vi "MC_7_13b_JW.vi"() -> ()   [LabVIEW 2011]
uses:
  <vilib>/Utility/file.llb/Read From Spreadsheet File (string).vi
  <vilib>/Utility/inputDevices.llb/keyboardAcquire.vi
  <vilib>/Utility/file.llb/Write To Spreadsheet File (DBL).vi
  <vilib>/Utility/file.llb/Write To Spreadsheet File (string).vi
  <vilib>/regexp/Match Regular Expression.xnode
panel:
  out "New: Temp":dbl
  out "XY Graph-Lin":cluster{dbl[], dbl[]}[](graph)
  out "Lin Vd":dbl
  out "Lin-Vg Array-Used":dbl[](array[numeric])
  out "Lin Id-Used":dbl[](array[numeric])
  out "Rec: Temp":dbl
  out "Comments":string
  out "Folder Index":dbl caption="Length"
  out "Current \nRecord":string[](array[string])
  out "Transformer \nHeaders":string[](array[string])
  out "Current Device ID":string
  out "Column":string
  out "Row":string
  out "Rec: Concentration":dbl
  out "Rec: Solvent":string
  out "Rec: Method":string
  in  "?":T1(tab)
  out "Rec: Material":string
  in  "Treatment Concentration (mM):":dbl=30.0
  in  "Surface Treatment:":string
  in  "# Drops*:":dbl=inf
  in  "Solution Temp (C):":dbl=55.0
  in  "Relative Humidity (%):":dbl=nan
  in  "Room Temp (F):":dbl=nan
  in  "Time (s):":dbl=80.0
  out "Accel (RPM/s):":dbl
  in  "RPM:":dbl=1000.0
  in  "Wait Time (s):":dbl=10.0
  in  "Sample #:":dbl=1.0
  in  "Fabricator:":string="Jeremy"
  in  "Data File":path
  out "Data Folder":path
  in  "Image Folder":path
  out "Image File":path=path "D:/UserData/Desktop/Jeremy/WFU/Research/Programs/VI mods/Image Not Found.png"
  in  "Ramp (s):":dbl=3.0
  in  "Manuel-Dielectric":bool
  in  "Manuel-Length":bool
  out "Calc: VT-Lin":dbl
  out "New: VT-Lin":dbl
  out "Rec: VT-Lin":dbl caption="VT-Lin" format="%#_3g"
  out "Calc: Trap Density-STS":dbl format="%#_4e"
  out "New: Trap Density-STS":dbl format="%#_4e"
  out "Rec: Trap Density-STS":dbl caption="N-Sat (STS)" format="%#_3e"
  out "Calc: Trap Density-VT":dbl format="%#_4e"
  out "New: Trap Density-VT":dbl format="%#_4e"
  out "Rec: Trap Density-VT":dbl caption="N-Sat (VT)" format="%#_3e"
  out "Calc: Mobility-Lin":dbl format="%#_4e"
  out "New: Mobility-Lin":dbl format="%#_4e"
  out "Rec: Mobility-Lin":dbl caption="Mobility-Lin" format="%#_3e"
  out "Calc: Mobility-Sat":dbl format="%#_4e"
  out "Rec: Length":dbl caption="Length" format="%#_3g"
  out "Rec: Width":dbl caption="Width" format="%#_4g"
  out "Rec: Dielectric (d)":dbl caption="Dielectric (d)" format="%#_3g"
  out "XY Graph":cluster{dbl[], dbl[]}[](graph)
  in  "NumPts":dbl=5.0
  in  "Cancel Button":bool
  in  "Next Button":bool
  in  "Previous Button":bool
  in  "Up Button":bool
  in  "Down Button":bool
  out "Data Name:":string
  in  "Save Changes?":bool
  in  "New: Dielectric":dbl
  in  "New: Length":dbl
  in  "New: Width":dbl
  out "New: Mobility-Sat":dbl format="%#_4e"
  in  "Slide":dbl(slide) step=1.0 scale=-14.3..88.0 scale format="%#_1p"
  in  "Blank Button":bool
  in  "Zoom":i16(slide)=-3 scale=-5.0..5.0
  out "Image Out 2":T2(plugin-control)
  out "Image Out":T2(plugin-control)
  in  "Magnification":u16(ring) items=["5x", "10x", "20x", "50x", "80x"]
  out "Total Width":dbl
  out "Distances":dbl[](array[numeric])
  in  "Undo Button":bool
  in  "Remove Button":bool
  out "Rec: Mobility-Sat":dbl caption="Mobility-Sat" format="%#_3e"
  out "Index":string
  out "Image Name":string
  in  "Export":bool
  out "Calc: VT-Sat":dbl
  out "New: VT-Sat":dbl
  in  "Manual-Width":bool caption="Manual"
  out "XY Graph 2":cluster{dbl[], dbl[]}[](graph)
  in  "Next Button 2":bool
  in  "Previous Button 2":bool
  in  "Slide 2":dbl(slide) step=1.0 scale=-1.0..82.0 scale format="%#_1p"
  out "Calc: STS":dbl
  out "New: STS":dbl
  in  "NumPts 2":dbl=5.0 caption="NumPts"
  out "Rec: VT-Sat":dbl caption="VT-Sat" format="%#_3g"
  out "Rec: STS":dbl caption="STS-Sat" format="%#_3g"
  out "Rec: On/Off":dbl caption="On/Off-Sat" format="%#_3e"
  in  "Save Changes? 2":bool
  in  "Save Changes? 3":bool
  out "Date Recorded":string="Date Recorded" caption="Recorded"
  out "Date Created":string caption="Fabricated"
  out "String":string
  in  "No Image":path=path "D:/UserData/Desktop/Jeremy/WFU/Research/Programs/VI mods/Image Not Found.png"
  in  "Project":path=path "D:/UserData/Desktop/Jeremy/WFU/Research/Programs/Mega Awesome/DeviceData.opj"
  out "Index 2":dbl
  out "Sat Id-Log-Used":dbl[](array[numeric])
  out "Vg Array-Log-Used":dbl[](array[numeric])
  out "ROI Descriptor out":T3 {"Contours"."Type" items=["No Selection", "Point", "Line", "Rectangle", "Oval", "Polygon", "Freehand Region", "Annulus", "Unused2", "Unused3", "Broken Line", "Freehand Line", "Rotated Rectangle"]}
  out "ROI Descriptor":T3 {"Contours"."Type" items=["No Selection", "Point", "Line", "Rectangle", "Oval", "Polygon", "Freehand Region", "Annulus", "Unused2", "Unused3", "Broken Line", "Freehand Line", "Rotated Rectangle"]}
  out "Numeric 3":dbl
  out "Array 6":dbl[][](array[numeric])
  out "Cluster":T4
  out "Array 5":dbl[](array[numeric])
  out "Array 4":dbl[](array[numeric])
  out "Array 3":dbl[](array[numeric])
  out "Numeric 2":dbl
  out "Numeric":dbl
  out "Sat Id-Used":dbl[](array[numeric])
  out "Sat Vg Array-Used":dbl[](array[numeric])
  out "MobVi Index":dbl
  in  "Row Start":dbl=20.0
  # "Data Locations"
  # "Data Location"
  # "Image Location"
  # "Sample Properties"
  # "*     Inf = Full coverage\n   NaN = Unknown or Not Applicable"
  # "Recorded"
  # "Calculated"
  # "Re-Calculated"
  # "Manual"
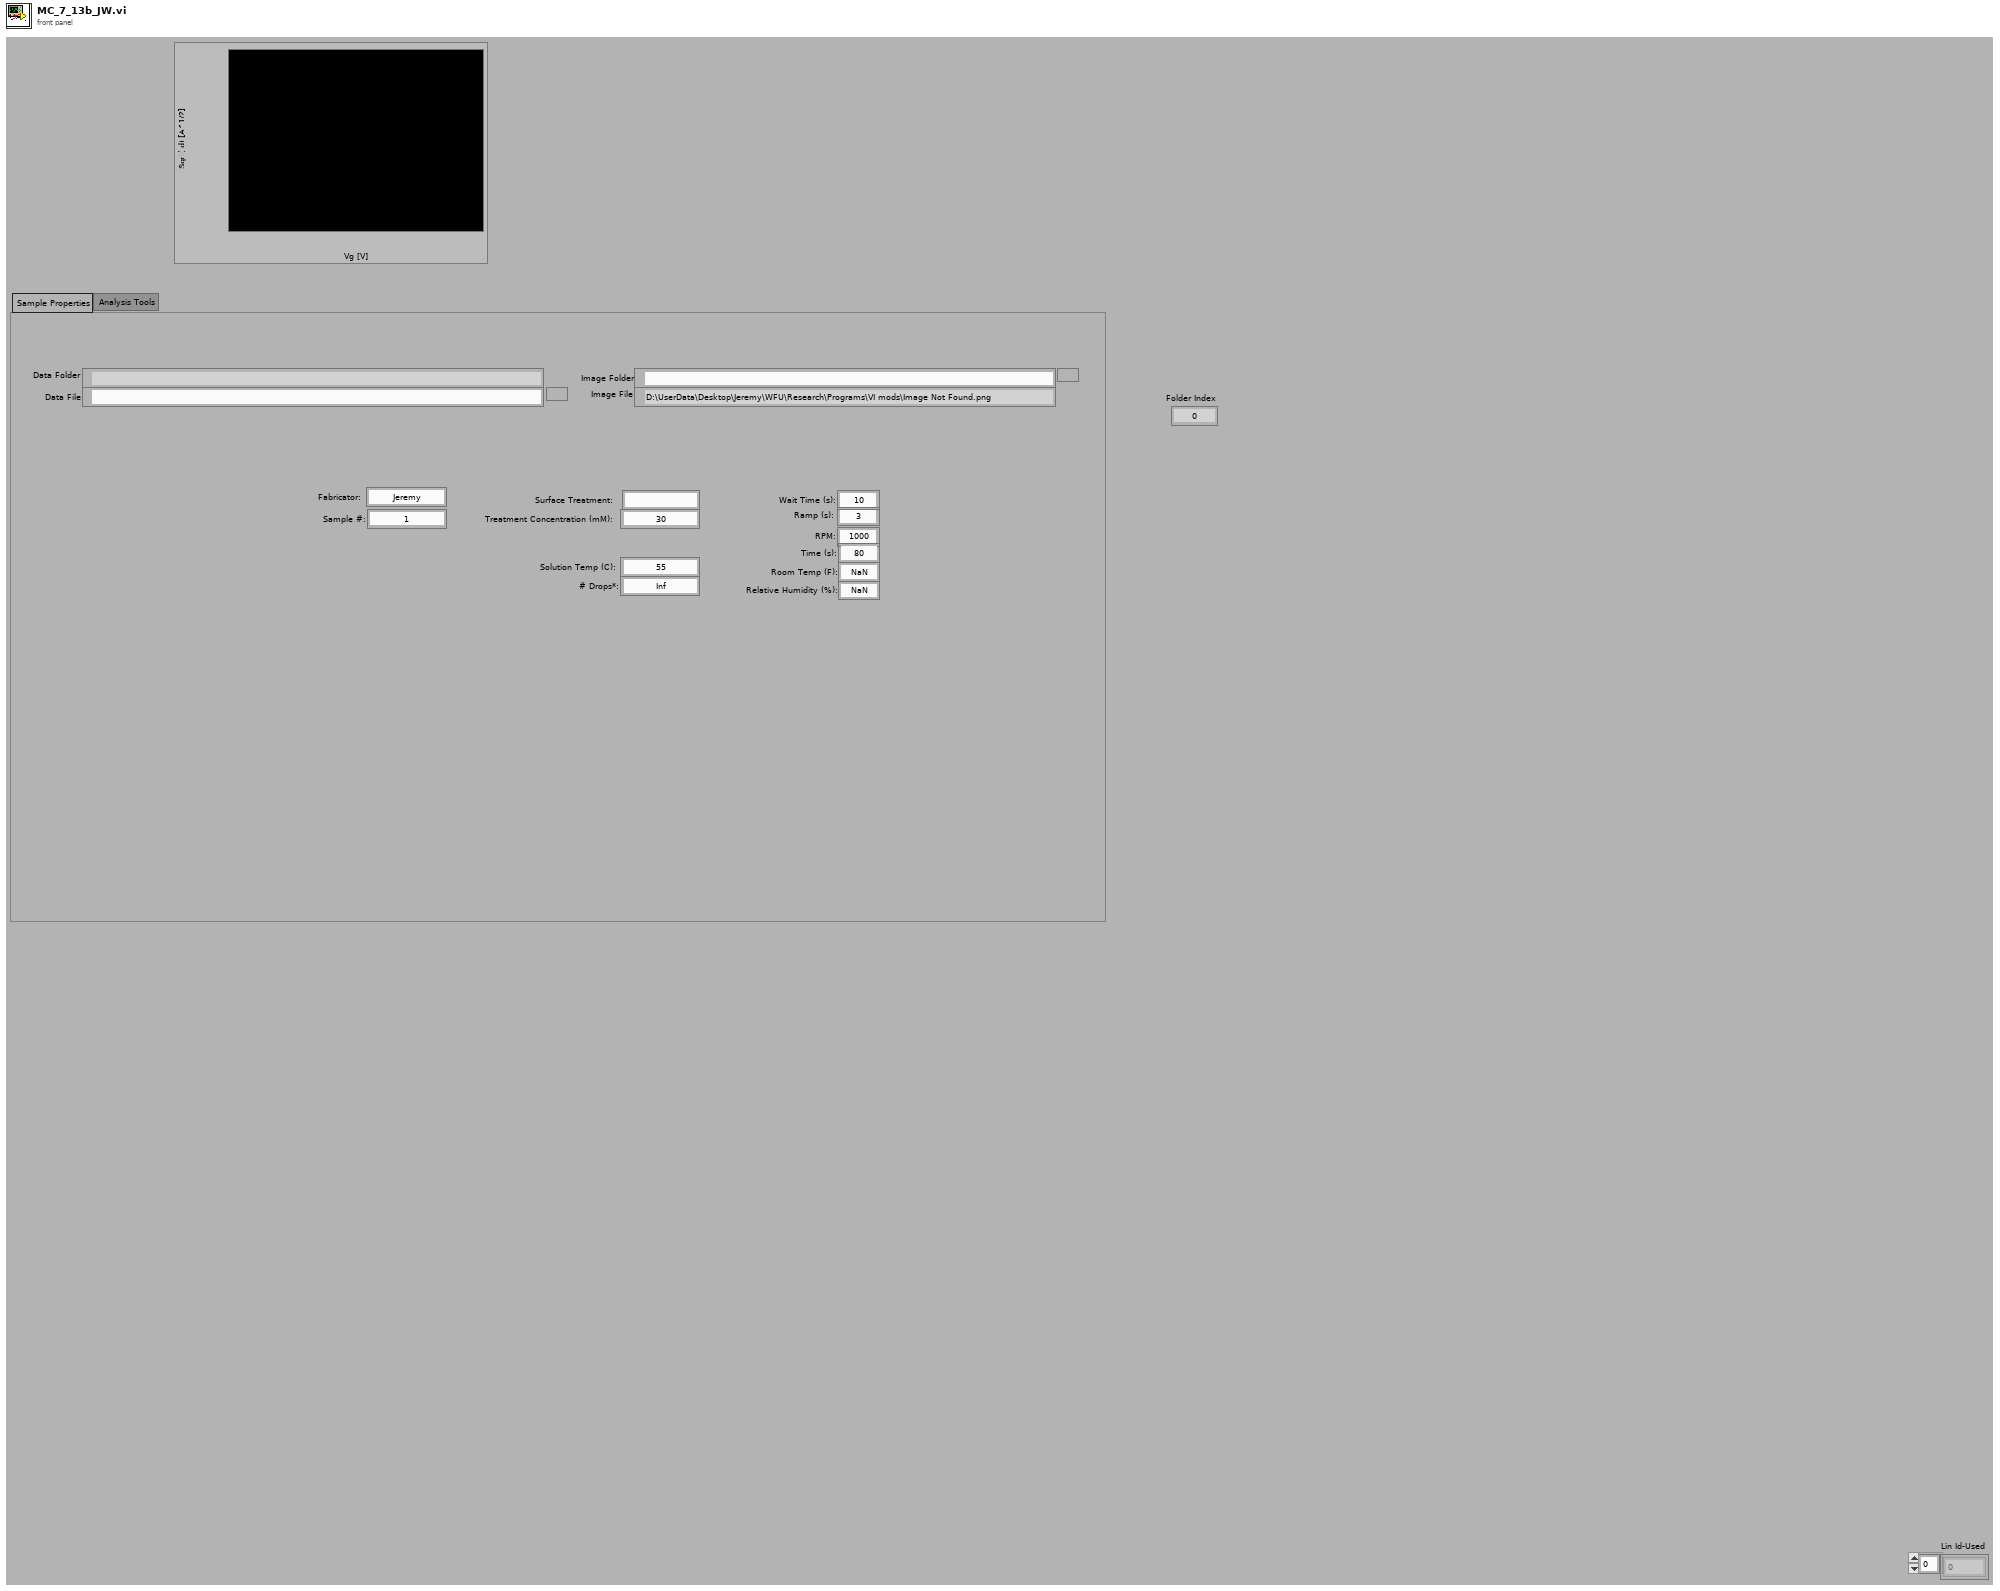
[diagram p1: front panel]
types:
  T1 = enum32{"Sample Properties", "Analysis Tools", "Current Database"}
  T2 = typedef "IMAQ Image.ctl" = refnum<image>
  T3 = typedef "ROI Descriptor" = cluster{"Global Rectangle":i32[], "Contours":cluster{"ID":enum32{"External", "Internal"}, "Type":u32, "Coordinates":i32[]}[]}
  T4 = cluster{"Numeric":dbl, "Numeric 2":dbl, "Numeric 3":dbl, "Numeric 4":dbl}
  T5 = cluster{"Mobility-Sat":dbl, "Moblitity-Lin":dbl, "On/Off":dbl, "Threshold Voltage":dbl, "Onset Voltage":dbl, "STS":dbl, "Trap Density-VT":dbl, "Trap Density-STS":dbl}
  T6 = cluster{"Date Recorded":string, "Index":string, "Length":dbl, "Width":dbl, "Sample Temp":dbl}
  T7 = cluster{"Date Created":string, "Material":string, "Solvent":string, "Concentration":dbl, "Method":string, "Dielectric (nm)":dbl, "Treatment":string, "Comments":string}
  T8 = cluster{"Mobility-Sat":dbl, "Vt-Sat":dbl, "Mobility-Lin":dbl, "Vt-Lin":dbl}
  T9 = cluster{"[0]":cluster{dbl[], dbl[]}, "[1]":cluster{dbl[], dbl[]}, "[2]":cluster{dbl[], dbl[]}, "[3]":cluster{dbl[], dbl[]}, "[4]":cluster{dbl[], dbl[]}, "[5]":cluster{dbl[], dbl[]}, "[6]":cluster{dbl[], dbl[]}, "[7]":cluster{dbl[], dbl[]}, "[8]":cluster{dbl[], dbl[]}}
  T10 = cluster{"Global Rectangle":i32[], "Contours":cluster{"Contour Type":u32, "ROI Type":u32, "Points":i32[]}[]}
  T11 = typedef "LVBoundsTypeDef.ctl" = cluster{"Width":u32, "Height":u32}
  T12 = enum16{"0", "1", "2", "3", "4", "5", "6", "7", "8", "9", "A", "B", "C", "D", "E", "F", "G", "H", "I", "J", "K", "L", "M", "N", "O", "P", "Q", "R", "S", "T", "U", "V", "W", "X", "Y", "Z", "F1", "F2", "F3", "F4", "F5", "F6", "F7", "F8", "F9", "F10", "F11", "F12", "F13", "F14", "F15", "ADD", "BACK", "BACKSLASH", "CAPITAL", "COMMA", "DECIMAL", "DELETE", "DIVIDE", "DOWN", "END", "EQUALS", "ESCAPE", "GRAVE (`)", "HOME", "INSERT", "LBRACKET", "LCONTROL", "LEFT", "L ALT", "LSHIFT", "LWIN", "MINUS", "MULTIPLY", "NEXT", "NUMLOCK", "NUMPAD_0", "NUMPAD_1", "NUMPAD_2", "NUMPAD_3", "NUMPAD_4", "NUMPAD_5", "NUMPAD_6", "NUMPAD_7", "NUMPAD_8", "NUMPAD_9", "PAUSE", "PERIOD", "PRIOR (PG UP)", "RBRACKET", "RCONTROL", "RETURN", "RIGHT", "R ALT", "RSHIFT", "RWIN", "SCROLL", "SEMICOLON", "SLASH", "SPACE", "SUBTRACT", "TAB", "UP", "ENTER (num pad)", "' (quote)"}[]
  T13 = enum16{"0", "1", "2", "3", "4", "5", "6", "7", "8", "9", "A", "B", "C", "D", "E", "F", "G", "H", "I", "J", "K", "L", "M", "N", "O", "P", "Q", "R", "S", "T", "U", "V", "W", "X", "Y", "Z", "F1", "F2", "F3", "F4", "F5", "F6", "F7", "F8", "F9", "F10", "F11", "F12", "F13", "F14", "F15", "ADD", "BACK", "BACKSLASH", "CAPITAL", "COMMA", "DECIMAL", "DELETE", "DIVIDE", "DOWN", "END", "EQUALS", "ESCAPE", "GRAVE (`)", "HOME", "INSERT", "LBRACKET", "LCONTROL", "LEFT", "L ALT", "LSHIFT", "LWIN", "MINUS", "MULTIPLY", "NEXT", "NUMLOCK", "NUMPAD_0", "NUMPAD_1", "NUMPAD_2", "NUMPAD_3", "NUMPAD_4", "NUMPAD_5", "NUMPAD_6", "NUMPAD_7", "NUMPAD_8", "NUMPAD_9", "PAUSE", "PERIOD", "PRIOR (PG UP)", "RBRACKET", "RCONTROL", "RETURN", "RIGHT", "R ALT", "RSHIFT", "RWIN", "SCROLL", "SEMICOLON", "SLASH", "SPACE", "SUBTRACT", "TAB", "UP", "ENTER (num pad)", "' (quote)"}
  T14 = cluster{"Contour Type":u32, "ROI Type":u32, "Points":i32[]}[]
  T15 = cluster{i32[], cluster{"Contour Type":u32, "ROI Type":u32, "Points":i32[]}[]}
  T16 = cluster{string, sgl, bool, bool, bool, bool, bool, bool, i32}
  T17 = cluster{i32, cluster{string, sgl, bool, bool, bool, bool, bool, bool, i32}, i32, i32}
  T18 = cluster{"Contour Type":u32, "ROI Type":u32, "Points":i32[]}
  T19 = cluster{"Points[0]":i32, "Points[1]":i32, "Points[2]":i32, "Points[3]":i32, "Points[4]":i32, "Points[5]":i32, "Points[6]":i32, "Points[7]":i32, "Points[8]":i32}
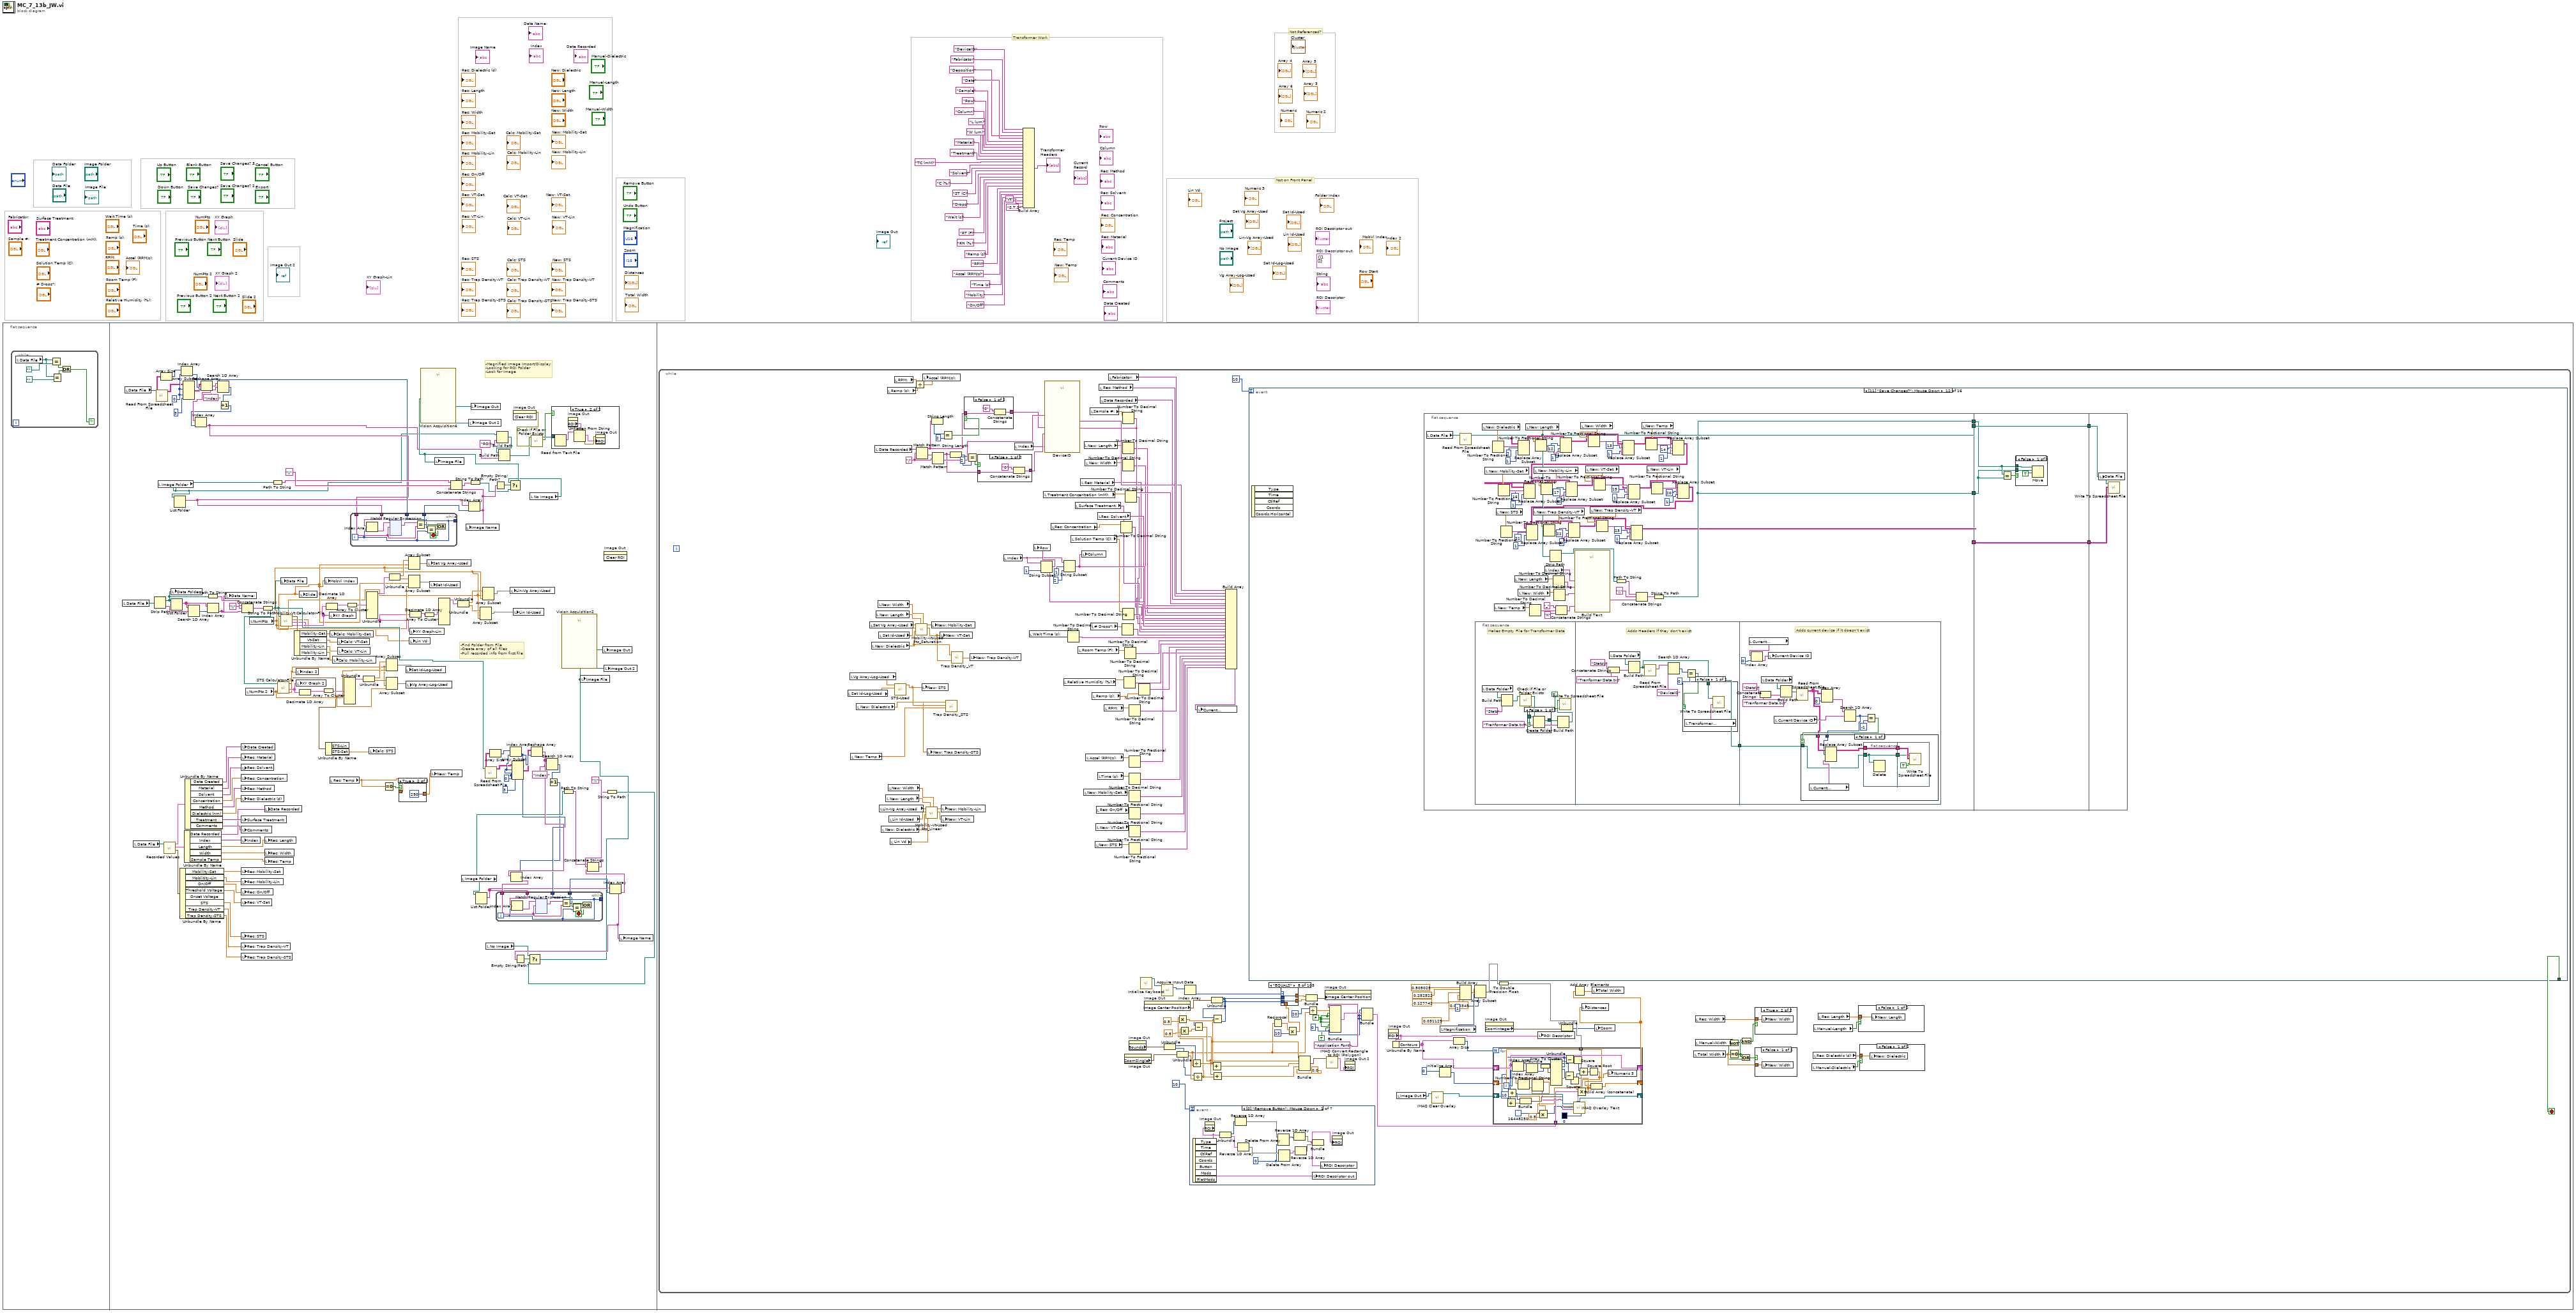
[diagram p0: block diagram]
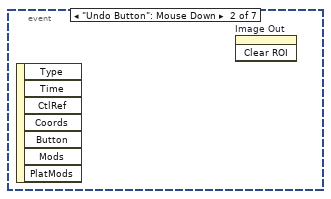
[diagram p10: hidden frame]
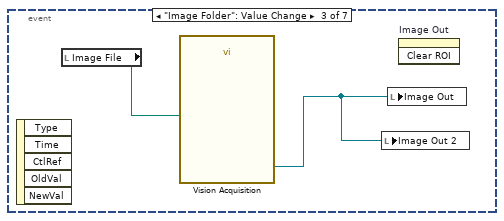
[diagram p11: hidden frame]
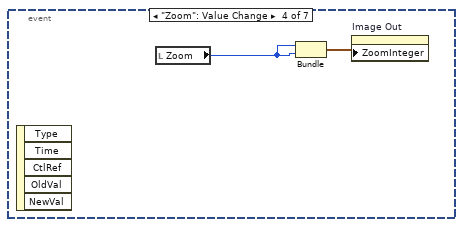
[diagram p12: hidden frame]
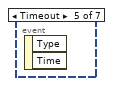
[diagram p13: hidden frame]
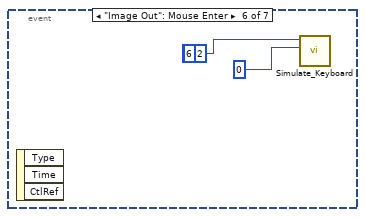
[diagram p14: hidden frame]
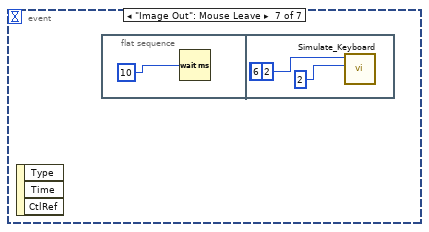
[diagram p15: hidden frame]
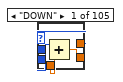
[diagram p16: hidden frame]
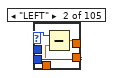
[diagram p17: hidden frame]
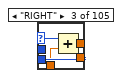
[diagram p18: hidden frame]
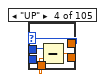
[diagram p19: hidden frame]
diagram:
  (unwired) T3 {"Global Rectangle"=[], "Contours"=[]}  # ROI Descriptor out
  # "Not Referenced?"
  # "Transformer Work"
  # "Not on Front Panel"
  n1 = flat-sequence {
    frame #0 {
      n2 = while {
        stop <- w29 continue-if-true
        n3 = local read "Data File"() -> (w31:path)
        n4 = Equal?(x=w31, y=path "") -> (x = y?=w33:bool)
        n5 = Equal?(x=w31, y=path "") -> (x = y?=w32:bool)
        n6 = Or(x=w33, y=w32) -> (x .or. y?=w29:bool)
      }
    }
    frame #1 {
      w126 = 0
      w150 = 0
      # "-Find Folder from File\n-Create array of all files\n-Pull recorded info from first file"
      # "-Magnified Image Import/Display\n-Looking for ROI Folder\n-Look for Image"
      n7 = local read "Data File"() -> (w130:path)
      n8 = local read "Data File"() -> (w145:path)
      n9 = local read "Data File"() -> (w85:path)
      n10 = Strip Path(path=w130) -> (stripped path=w131:path, name=w117:string)
      n11 = call-poly <vilib>:"Read From Spreadsheet File.vi"("file path (dialog if empty)"=w145) -> ("all rows"=w148:string[][])  [unwired: 6 in, 4 out]
      n12 = local read "Image Folder"() -> (w87:path)
      n13 = Array Size(array=w148) -> (size(s)=w149:i32[])
      n14 = call "Recorded Values.vi"("Path"=w85) -> ("Recorded Char"=w83:T5, "Recorded Prop"=w82:T6, "Fabrication Prop"=w84:T7)  [unwired: 8 in]
      n15 = local write "Data Folder"(w131) -> ()
      n16 = List Folder(path=w131) -> (filenames=w121:string[])  [unwired: 3 in, 3 out]
      n17 = List Folder(path=w87) -> (filenames=w154:string[])  [unwired: 3 in, 3 out]
      n18 = Unbundle By Name(w83) -> ("Mobility-Sat"=w69:dbl, "Moblitity-Lin"=w68:dbl, "On/Off"=w67:dbl, "Threshold Voltage"=w66:dbl, "STS"=w65:dbl, "Trap Density-VT"=w64:dbl, "Trap Density-STS"=w63:dbl)  [unwired: 1 out]
      n19 = Index Array(array=w149, index=w150) -> (element=w156:i32)
      n20 = Array Subset(array=w148, index (row)=w150, index (col)=w150, length (col)=3) -> (w147:string[][])  [unwired: 1 in]
      n21 = Unbundle By Name(w82) -> ("Date Recorded"=w74:string, "Index"=w73:string, "Length"=w72:dbl, "Width"=w71:dbl, "Sample Temp"=w70:dbl)
      n22 = Unbundle By Name(w84) -> ("Date Created"=w62:string, "Material"=w81:string, "Solvent"=w80:string, "Concentration"=w79:dbl, "Method"=w78:string, "Dielectric (nm)"=w77:dbl, "Treatment"=w76:string, "Comments"=w75:string)
      n23 = Search 1D Array(1D array=w121, element=w117) -> (index of element=w120:i32)  [unwired: 1 in]
      n24 = Reshape Array(w147, w156) -> (w161:string[])
      n25 = Path To String(path=w131) -> (string=w116:string)
      n26 = Index Array(array=w121, index=w120) -> (element=w86:string)
      n27 = Search 1D Array(1D array=w161, element="Index:") -> (index of element=w153:i32)  [unwired: 1 in]
      n28 = Increment(x=w153) -> (x+1=w152:i32)
      n29 = Index Array(array=w161, index=w152) -> (element=w88:string)
      n30 = local write "Data Name:"(w86) -> ()
      n31 = local write "Date Created"(w62) -> ()
      n32 = local write "Rec: Material"(w81) -> ()
      n33 = local write "Rec: Solvent"(w80) -> ()
      n34 = local write "Rec: Concentration"(w79) -> ()
      n35 = local write "Rec: Method"(w78) -> ()
      n36 = local write "Rec: Dielectric (d)"(w77) -> ()
      n37 = local write "Surface Treatment:"(w76) -> ()
      n38 = local write "Comments"(w75) -> ()
      n39 = local write "Index"(w73) -> ()
      n40 = local write "Rec: Mobility-Sat"(w69) -> ()
      n41 = local write "Rec: Mobility-Lin"(w68) -> ()
      n42 = local write "Rec: On/Off"(w67) -> ()
      n43 = local write "Rec: VT-Sat"(w66) -> ()
      n44 = local write "Rec: STS"(w65) -> ()
      n45 = local write "Rec: Trap Density-VT"(w64) -> ()
      n46 = local write "Rec: Trap Density-STS"(w63) -> ()
      n47 = Concatenate Strings(w116, "\\", w86) -> (w118:string)
      n48 = local read "NumPts 2"() -> (w53:dbl)
      n49 = local read "NumPts"() -> (w43:dbl)
      n50 = String To Path(string=w118) -> (path=w61:path)
      n51 = local write "Date Recorded"(w74) -> ()
      n52 = local write "Rec: Length"(w72) -> ()
      n53 = local write "Rec: Width"(w71) -> ()
      n54 = local write "Rec: Temp"(w70) -> ()
      n55 = Path To String(path=w87) -> (string=w158:string)
      n56 = call "STS Calculator-File.vi"("NumPts"=w53, "Path"=w61) -> ("STS Index-Sat"=w51:dbl, "XY Graph-Sat"=w52:cluster{dbl[], dbl[]}[], "Ouput"=w50:cluster{"STS-Sat":dbl, "STS-Lin":dbl})  [unwired: 5 in, 2 out]
      n57 = local write "Data File"(w61) -> ()
      n58 = call "Mobility-Vt Calculator-File.vi"("NumPts"=w43, "Path"=w61) -> ("XY Graph-Sat"=w55:cluster{dbl[], dbl[]}[], "XY Graph-Lin"=w38:cluster{dbl[], dbl[]}[], "Lin Vd"=w39:dbl, "Output"=w56:T8, "Index-Sat"=w54:dbl, "Index-Lin"=w42:dbl)  [unwired: 4 in]
      n59 = Unbundle By Name(w56) -> ("Mobility-Sat"=w60:dbl, "Vt-Sat"=w59:dbl, "Mobility-Lin"=w58:dbl, "Mobility-Lin"=w57:dbl)
      n60 = local write "Index 2"(w51) -> ()
      n61 = local write "XY Graph 2"(w52) -> ()
      n62 = local write "Slide"(w54) -> ()
      n63 = Decimate 1D Array(w52) -> (w108:cluster{dbl[], dbl[]}[])  [unwired: 1 out]
      n64 = Array To Cluster(array=w108) -> (cluster=w110:T9)
      n65 = local write "MobVi Index"(w54) -> ()
      n66 = Unbundle By Name(w50) -> ("STS-Sat"=w49:dbl)  [unwired: 1 out]
      n67 = Decimate 1D Array(w55) -> (w144:cluster{dbl[], dbl[]}[])  [unwired: 1 out]
      n68 = local write "XY Graph"(w55) -> ()
      n69 = local read "Rec: Temp"() -> (w36:dbl)
      n70 = local write "Calc: Mobility-Sat"(w60) -> ()
      n71 = local write "Calc: Mobility-Lin"(w57) -> ()
      n72 = local write "Calc: VT-Sat"(w59) -> ()
      n73 = local write "Calc: VT-Lin"(w58) -> ()
      n74 = Unbundle(w110) -> ("[0]"=w109:cluster{dbl[], dbl[]})  [unwired: 8 out]
      n75 = Array To Cluster(array=w144) -> (cluster=w142:T9)
      n76 = while {
        tunnel: w154 -> [w296]
        tunnel: w88 -> [w294]
        tunnel: [w293] -> _
        tunnel: [w293] -> w155
        tunnel: w156 -> [w292]
        i -> [w293]
        stop <- w289 stop-if-true
        n77 = Index Array(array=w296, index=w293) -> (element=w297:string)
        n78 = xnode "Match Regular Expression"("input string"=w297, "regular expression"=w294) -> ("whole match"=w295:string)  [unwired: 4 in, 4 out]
        n79 = Equal?(x=w295, y=w294) -> (x = y?=w291:bool)
        n80 = Equal?(x=w292, y=w293) -> (x = y?=w290:bool)
        n81 = Or(x=w291, y=w290) -> (x .or. y?=w289:bool)
      }
      n82 = Unbundle(w109) -> (w106:dbl[], w105:dbl[])
      n83 = Unbundle(w142) -> ("[0]"=w143:cluster{dbl[], dbl[]})  [unwired: 8 out]
      n84 = local write "Calc: STS"(w49) -> ()
      n85 = Equal To 0?(x=w36) -> (x = 0?=w37:bool)
      n86 = Array Subset(array=w106, index=w51, length=w53) -> (w113:dbl[])
      n87 = Array Subset(array=w105, index=w51, length=w53) -> (w112:dbl[])
      n88 = Unbundle(w143) -> (w107:dbl[], w111:dbl[])
      n89 = case shown="True" w37 {
        tunnel: [w162 290] -> w35
        tunnel: w36 -> [w162 _]
        frame False {
        }
        frame True {
        }
      }
      n90 = local write "Sat Id-Log-Used"(w113) -> ()
      n91 = local write "Vg Array-Log-Used"(w112) -> ()
      n92 = Array Subset(array=w107, index=w54, length=w43) -> (w114:dbl[])
      n93 = Array Subset(array=w111, index=w54, length=w43) -> (w115:dbl[])
      n94 = local write "Lin Vd"(w39) -> ()
      n95 = Decimate 1D Array(w38) -> (w48:cluster{dbl[], dbl[]}[])  [unwired: 1 out]
      n96 = local write "XY Graph-Lin"(w38) -> ()
      n97 = Array To Cluster(array=w48) -> (cluster=w47:T9)
      n98 = local write "Sat Vg Array-Used"(w114) -> ()
      n99 = local write "Sat Id-Used"(w115) -> ()
      n100 = local write "New: Temp"(w35) -> ()
      n101 = Unbundle(w47) -> ("[0]"=w46:cluster{dbl[], dbl[]})  [unwired: 8 out]
      n102 = Unbundle(w46) -> (w45:dbl[], w44:dbl[])
      n103 = local read "Image Folder"() -> (w137:path)
      n104 = Index Array(array=w154, index=w155) -> (element=w104:string)
      n105 = Concatenate Strings(w158, "\\", w104) -> (w159:string)
      n106 = local write "Image Name"(w104) -> ()
      n107 = String To Path(string=w159) -> (path=w102:path)
      n108 = List Folder(path=w137) -> (filenames=w133:string[])  [unwired: 3 in, 3 out]
      n109 = Array Subset(array=w44, index=w42, length=w43) -> (w40:dbl[])
      n110 = Array Subset(array=w45, index=w42, length=w43) -> (w41:dbl[])
      n111 = call-poly <vilib>:"Read From Spreadsheet File.vi"("file path (dialog if empty)"=w61) -> ("all rows"=w124:string[][])  [unwired: 6 in, 4 out]
      n112 = local read "No Image"() -> (w96:path)
      n113 = Array Size(array=w124) -> (size(s)=w125:i32[])
      n114 = Empty String/Path?(string/path=w104) -> (empty?=w103:bool)
      n115 = Build Path(base path=w87, name or relative path="ROI") -> (appended path=w90:path)
      n116 = Build Path(base path=w90, name or relative path=w88) -> (appended path=w89:path)
      n117 = Index Array(array=w125, index=w126) -> (element=w136:i32)
      n118 = local write "Lin-Vg Array-Used"(w41) -> ()
      n119 = Array Subset(array=w124, index (row)=w126, index (col)=w126, length (col)=3) -> (w123:string[][])  [unwired: 1 in]
      n120 = local write "Lin Id-Used"(w40) -> ()
      n121 = invoke on="Image Out" class="ImageControl" method="Clear ROI"() -> (error out=w94:errorcluster)  [unwired: 3 in, 2 out]
      n122 = local read "No Image"() -> (w95:path)
      n123 = Select(t=w95, s=w103, f=w102) -> (s? t:f=w101:path)
      n124 = call "Vision Acquisition6"("Image Path"=w101) -> ("Image Out"=w157:T2)  [unwired: 25 in, 1 out]
      n125 = local write "Image File"(w101) -> ()
      n126 = local write "Image Out 2"(w157) -> ()
      n127 = local write "Image Out"(w157) -> ()
      n128 = call <vilib>:"Check if File or Folder Exists.vi"("error in (no error)"=w94, "path"=w89) -> ("file or folder exists?"=w92:bool, "dup path"=w93:path)  [unwired: 7 in, 1 out]
      n129 = Reshape Array(w123, w136) -> (w141:string[])
      n130 = Search 1D Array(1D array=w141, element="Index:") -> (index of element=w129:i32)  [unwired: 1 in]
      n131 = Increment(x=w129) -> (x+1=w128:i32)
      n132 = Index Array(array=w141, index=w128) -> (element=w134:string)
      n133 = while {
        tunnel: w133 -> [w176]
        tunnel: w134 -> [w174]
        tunnel: [w173] -> _
        tunnel: [w173] -> w135
        tunnel: w136 -> [w172]
        i -> [w173]
        stop <- w169 stop-if-true
        n134 = Index Array(array=w176, index=w173) -> (element=w177:string)
        n135 = xnode "Match Regular Expression"("input string"=w177, "regular expression"=w174) -> ("whole match"=w175:string)  [unwired: 4 in, 4 out]
        n136 = Equal?(x=w175, y=w174) -> (x = y?=w171:bool)
        n137 = Equal?(x=w172, y=w173) -> (x = y?=w170:bool)
        n138 = Or(x=w171, y=w170) -> (x .or. y?=w169:bool)
      }
      n139 = case shown="True" w92 {
        tunnel: w93 -> [_ w164]
        frame False {
        }
        frame True {
          n140 = Read from Text File(file (use dialog)=w164) -> (text=w168:string)  [unwired: 3 in, 3 out]
          n141 = property on="Image Out" class="ImageControl"() -> ("ROI"=w165:T10)  [unwired: 2 in, 2 out]
          n142 = Unflatten From String(type=w165, binary string=w168) -> (value=w166:T10, error out=w167:errorcluster)  [unwired: 3 in, 1 out]
          n143 = property on="Image Out" class="ImageControl"(error in=w167, "ROI"=w166) -> ()  [unwired: 1 in, 2 out]
        }
      }
      n144 = Path To String(path=w137) -> (string=w138:string)
      n145 = invoke on="Image Out" class="ImageControl" method="Clear ROI"() -> ()  [unwired: 3 in, 3 out]
      n146 = Index Array(array=w133, index=w135) -> (element=w99:string)
      n147 = Empty String/Path?(string/path=w99) -> (empty?=w100:bool)
      n148 = Concatenate Strings(w138, "\\", w99) -> (w139:string)
      n149 = String To Path(string=w139) -> (path=w98:path)
      n150 = Select(t=w96, s=w100, f=w98) -> (s? t:f=w97:path)
      n151 = call "Vision Acquisition2"("Image Path"=w97) -> ("Image Out"=w132:T2)  [unwired: 25 in, 1 out]
      n152 = local write "Image File"(w97) -> ()
      n153 = local write "Image Out"(w132) -> ()
      n154 = local write "Image Out 2"(w132) -> ()
      n155 = local write "Image Name"(w99) -> ()
    }
    frame #2 {
      n156 = while {
        stop <- w572 stop-if-true
        w468 = "/"
        w522 = FALSE
        w520 = 0
        n157 = local read "Sat Id-Log-Used"() -> (w425:dbl[])
        n158 = local read "Vg Array-Log-Used"() -> (w424:dbl[])
        n159 = local read "New: Temp"() -> (w409:dbl)
        n160 = local read "New: Dielectric"() -> (w414:dbl)
        n161 = local read "Sat Vg Array-Used"() -> (w427:dbl[])
        n162 = local read "New: Dielectric"() -> (w411:dbl)
        n163 = local read "Date Recorded"() -> (w471:string)
        n164 = local read "New: Length"() -> (w428:dbl)
        n165 = local read "New: Width"() -> (w430:dbl)
        n166 = local read "Sat Id-Used"() -> (w426:dbl[])
        n167 = local read "Lin-Vg Array-Used"() -> (w421:dbl[])
        n168 = local read "New: Dielectric"() -> (w418:dbl)
        n169 = local read "New: Length"() -> (w420:dbl)
        n170 = local read "Ramp (s):"() -> (w438:dbl)
        n171 = local read "New: Width"() -> (w417:dbl)
        n172 = local read "Lin Id-Used"() -> (w422:dbl[])
        n173 = local read "Lin Vd"() -> (w416:dbl)
        n174 = local read "RPM:"() -> (w439:dbl)
        n175 = call "STS-Used.vi"("Id Used"=w425, "Vg-Used"=w424) -> ("STS"=w415:dbl)  [unwired: 9 in]
        n176 = Divide(x=w439, y=w438) -> (x/y=w437:dbl)
        n177 = call "Mobility-Vt-Used Pts_Saturation.vi"("Width"=w430, "Length"=w428, "Dielectric (d)"=w411, "Sat Id Used"=w426, "Vg Used"=w427) -> ("Vt"=w412:dbl, "Mobility"=w429:dbl)  [unwired: 4 in, 1 out]
        n178 = Match Pattern(string=w471, regular expression=w468) -> (before substring=w462:string, after substring=w469:string)  [unwired: 1 in, 2 out]
        n179 = local write "New: STS"(w415) -> ()
        n180 = local write "Accel (RPM/s):"(w437) -> ()
        n181 = call "Mobility-Vt-Used Pts_Linear.vi"("Width"=w417, "Length"=w420, "Vd"=w416, "Dielectric (d)"=w418, "Sat Id Used"=w422, "Vg Used"=w421) -> ("Vt"=w423:dbl, "Mobility"=w419:dbl)  [unwired: 3 in, 1 out]
        n182 = String Length(string=w462) -> (length=w465:i32)
        n183 = local write "New: Mobility-Sat"(w429) -> ()
        n184 = Match Pattern(string=w469, regular expression=w468) -> (before substring=w456:string, after substring=w467:string)  [unwired: 1 in, 2 out]
        n185 = local write "New: VT-Sat"(w412) -> ()
        n186 = local write "New: Mobility-Lin"(w419) -> ()
        n187 = local write "New: VT-Lin"(w423) -> ()
        n188 = Equal?(x=w465, y=2) -> (x = y?=w463:bool)
        n189 = call "Trap Density_STS.vi"("Temp (T) [K]"=w409, "S.T.S. (S)"=w415, "Dielectric"=w414) -> ("Trap Density (N)"=w413:dbl)  [unwired: 8 in]
        n190 = local write "New: Trap Density-STS"(w413) -> ()
        n191 = String Length(string=w456) -> (length=w458:i32)
        n192 = call "Trap Density_VT.vi"("VT"=w412, "Dielectric"=w411) -> ("Trap Density-VT"=w410:dbl)
        n193 = case shown="False" w463 {
          tunnel: w462 -> [w580 w582]
          tunnel: [w579 w582] -> w461
          frame False {
            n194 = Concatenate Strings("0", w580) -> (w579:string)
          }
          frame True {
          }
        }
        n195 = Equal?(x=w458, y=2) -> (x = y?=w460:bool)
        n196 = local write "New: Trap Density-VT"(w410) -> ()
        n197 = case shown="False" w460 {
          tunnel: w456 -> [w576 w578]
          tunnel: [w575 w578] -> w457
          frame False {
            n198 = Concatenate Strings("0", w576) -> (w575:string)
          }
          frame True {
          }
        }
        n199 = local read "Index"() -> (w441:string)
        n200 = local read "Index"() -> (w455:string)
        n201 = local read "Wait Time (s):"() -> (w501:dbl)
        n202 = String Subset(string=w441, length (rest)=1) -> (substring=w496:string)  [unwired: 1 in]
        n203 = local write "Row"(w496) -> ()
        n204 = local read "Treatment Concentration (mM):"() -> (w449:dbl)
        n205 = local read "Rec: Concentration"() -> (w436:dbl)
        n206 = local read "Relative Humidity (%):"() -> (w446:dbl)
        n207 = String Subset(string=w441, offset (0)=1, length (rest)=2) -> (substring=w497:string)
        n208 = Number To Decimal String(number=w501) -> (decimal integer string=w502:string)  [unwired: 1 in]
        n209 = local read "Solution Temp (C):"() -> (w490:dbl)
        n210 = local read "Surface Treatment:"() -> (w448:string)
        n211 = local read "Room Temp (F):"() -> (w494:dbl)
        n212 = local read "Rec: Material"() -> (w444:string)
        n213 = local write "Column"(w497) -> ()
        n214 = local read "New: Mobility-Sat"() -> (w483:dbl)
        n215 = local read "New: Length"() -> (w454:dbl)
        n216 = local read "New: Width"() -> (w453:dbl)
        n217 = local read "Accel (RPM/s):"() -> (w481:dbl)
        n218 = local read "Sample #:"() -> (w473:dbl)
        n219 = local read "# Drops*:"() -> (w491:dbl)
        n220 = local read "Ramp (s):"() -> (w499:dbl)
        n221 = local read "New: STS"() -> (w475:dbl)
        n222 = local read "New: VT-Sat"() -> (w477:dbl)
        n223 = local read "Rec: On/Off"() -> (w479:dbl)
        n224 = local read "Rec: Solvent"() -> (w450:string)
        n225 = local read "Time (s):"() -> (w486:dbl)
        n226 = local read "Rec: Method"() -> (w474:string)
        n227 = local read "Date Recorded"() -> (w470:string)
        n228 = local read "RPM:"() -> (w487:dbl)
        n229 = local read "Fabricator:"() -> (w495:string)
        n230 = Number To Decimal String(number=w436) -> (decimal integer string=w435:string)  [unwired: 1 in]
        n231 = Number To Decimal String(number=w491) -> (decimal integer string=w492:string)  [unwired: 1 in]
        n232 = Number To Decimal String(number=w473) -> (decimal integer string=w466:string)  [unwired: 1 in]
        n233 = call "DeviceID"("Sample"=w466, "Year"=w467, "Month"=w461, "Day"=w457, "Index"=w455) -> ("Result"=w472:string)  [unwired: 9 in, 1 out]
        n234 = Number To Decimal String(number=w454) -> (decimal integer string=w452:string)  [unwired: 1 in]
        n235 = Number To Decimal String(number=w453) -> (decimal integer string=w451:string)  [unwired: 1 in]
        n236 = Number To Decimal String(number=w490) -> (decimal integer string=w489:string)  [unwired: 1 in]
        n237 = Number To Decimal String(number=w446) -> (decimal integer string=w445:string)  [unwired: 1 in]
        n238 = Number To Decimal String(number=w494) -> (decimal integer string=w493:string)  [unwired: 1 in]
        n239 = property on="Image Out" class="ImageControl"() -> ("ZoomSingle"=w540:cluster{"X":sgl, "Y":sgl})  [unwired: 2 in, 2 out]
        n240 = Number To Decimal String(number=w449) -> (decimal integer string=w447:string)  [unwired: 1 in]
        n241 = property on="Image Out" class="ImageControl"() -> ("Bounds"=w541:T11)  [unwired: 2 in, 2 out]
        n242 = Number To Decimal String(number=w487) -> (decimal integer string=w488:string)  [unwired: 1 in]
        n243 = Number To Fractional String(number=w481) -> (F-format string=w482:string)  [unwired: 3 in]
        n244 = Number To Decimal String(number=w486) -> (decimal integer string=w485:string)  [unwired: 1 in]
        n245 = Number To Fractional String(number=w483) -> (F-format string=w484:string)  [unwired: 3 in]
        n246 = Number To Fractional String(number=w479) -> (F-format string=w480:string)  [unwired: 3 in]
        n247 = Number To Fractional String(number=w477) -> (F-format string=w478:string)  [unwired: 3 in]
        n248 = Number To Fractional String(number=w475) -> (F-format string=w476:string)  [unwired: 3 in]
        n249 = Number To Decimal String(number=w499) -> (decimal integer string=w500:string)  [unwired: 1 in]
        n250 = call <vilib>:"Intialize Keyboard.vi"() -> ("device ID"=w552:refnum<k1>)  [unwired: 10 in, 1 out]
        n251 = property on="Image Out" class="ImageControl"() -> ("Image Center Position"=w547:cluster{"X":u32, "Y":u32})  [unwired: 2 in, 2 out]
        n252 = call-poly <vilib>:"Acquire Input Data.vi"("device ID"=w552) -> ("keys pressed"=w551:T12)  [unwired: 16 in, 2 out]
        n253 = Unbundle(w541) -> ("Width"=w538:u32, "Height"=w537:u32)
        n254 = Unbundle(w540) -> ("X"=w515:sgl, "Y"=w539:sgl)
        n255 = Index Array(array=w551) -> (element=w555:T13)  [unwired: 1 in]
        n256 = event shown="[0] \"Remove Button\": Mouse Down" {
          selector: _ -> [_ _ _ _ _ _ _]
          dyn-events: _ -> [_ _ _ _ _ _ _]
          timeout: 10 -> [_ _ _ _ _ _ _]
          event "Remove Button": Mouse Down {
            w587 = 0
            n257 = event-data() -> ()  [unwired: 1 in, 7 out]
            n258 = property on="Image Out" class="ImageControl"() -> ("ROI"=w585:T10)  [unwired: 2 in, 2 out]
            n259 = Unbundle(w585) -> ("Global Rectangle"=w588:i32[], "Contours"=w590:T14)
            n260 = Reverse 1D Array(array=w588) -> (reversed array=w589:i32[])
            n261 = Reverse 1D Array(array=w590) -> (reversed array=w591:T14)
            n262 = Delete From Array(array=w589, index=w587) -> (array with subset deleted=w592:i32[])  [unwired: 1 in, 1 out]
            n263 = Delete From Array(array=w591, index=w587) -> (array with subset deleted=w593:T14)  [unwired: 1 in, 1 out]
            n264 = Reverse 1D Array(array=w592) -> (reversed array=w594:i32[])
            n265 = Reverse 1D Array(array=w593) -> (reversed array=w595:T14)
            n266 = Bundle(w594, w595) -> (w586:T15)  [unwired: 1 in]
            n267 = local write "ROI Descriptor out"(w585) -> ()
            n268 = local write "ROI Descriptor"(w586) -> ()
            n269 = property on="Image Out" class="ImageControl"("ROI"=w586) -> ()  [unwired: 2 in, 2 out]
          }
          event "Undo Button": Mouse Down {
            n270 = event-data() -> ()  [unwired: 1 in, 7 out]
            n271 = invoke on="Image Out" class="ImageControl" method="Clear ROI"() -> ()  [unwired: 3 in, 3 out]
          }
          event "Image Folder": Value Change {
            n272 = event-data() -> ()  [unwired: 1 in, 5 out]
            n273 = local read "Image File"() -> (w597:path)
            n274 = call "Vision Acquisition"("Image Path"=w597) -> ("Image Out"=w596:T2)  [unwired: 25 in, 1 out]
            n275 = local write "Image Out 2"(w596) -> ()
            n276 = local write "Image Out"(w596) -> ()
            n277 = invoke on="Image Out" class="ImageControl" method="Clear ROI"() -> ()  [unwired: 3 in, 3 out]
          }
          event "Zoom": Value Change {
            n278 = event-data() -> ()  [unwired: 1 in, 5 out]
            n279 = local read "Zoom"() -> (w598:i16)
            n280 = Bundle("Zoom"=w598, "Zoom"=w598) -> (w599:cluster{"Zoom":i16, "Zoom":i16})  [unwired: 1 in]
            n281 = property on="Image Out" class="ImageControl"("ZoomInteger"=w599) -> ()  [unwired: 2 in, 2 out]
          }
          event Timeout {
            n282 = event-data() -> ()  [unwired: 1 in, 2 out]
          }
          event "Image Out": Mouse Enter {
            (unwired) 6
            n283 = event-data() -> ()  [unwired: 1 in, 3 out]
            n284 = call "Simulate_Keyboard.vi"("Action"=0, "Virtual Key"=162) -> ()  [unwired: 7 in, 1 out]
          }
          event "Image Out": Mouse Leave {
            n285 = event-data() -> ()  [unwired: 1 in, 3 out]
            n286 = flat-sequence {
              frame #0 {
                n287 = Wait (ms)(milliseconds to wait=10) -> ()  [unwired: 1 out]
              }
              frame #1 {
                (unwired) 6
                n288 = call "Simulate_Keyboard.vi"("Action"=2, "Virtual Key"=162) -> ()  [unwired: 7 in, 1 out]
              }
            }
          }
        }
        n289 = Divide(x=w538, y=w515) -> (x/y=w528:sgl)
        n290 = Multiply(x=w528, y=0.5) -> (x*y=w534:dbl)
        n291 = Divide(x=w537, y=w539) -> (x/y=w527:sgl)
        n292 = Multiply(x=w527, y=0.5) -> (x*y=w533:dbl)
        n293 = Unbundle(w547) -> ("X"=w529:u32, "Y"=w530:u32)
        n294 = Subtract(x=w530, y=w533) -> (x-y=w531:dbl)
        n295 = Subtract(x=w529, y=w534) -> (x-y=w532:dbl)
        n296 = Add(x=w532, y=w528) -> (x+y=w546:dbl)
        n297 = Add(x=w531, y=w527) -> (x+y=w545:dbl)
        n298 = Build Array(w472, w495, w474, w470, w466, w496, w497, w452, w451, w444, w448, w447, w450, w435, w489, w492, w502, w493, w445, w500, w488, w482, w485, w484, w480, w478, w476) -> (w498:string[])
        n299 = local write "Current \nRecord"(w498) -> ()
        n300 = event shown="[11] \"Save Changes?\": Mouse Down" {
          selector: _ -> [_ _ _ _ _ _ _ _ _ _ _ _ _ _ _ _]
          dyn-events: _ -> [_ _ _ _ _ _ _ _ _ _ _ _ _ _ _ _]
          timeout: 10 -> [_ _ _ _ _ _ _ _ _ _ _ _ _ _ _ _]
          tunnel: [_ _ _ _ _ _ _ _ _ _ _ _ _ TRUE _ TRUE] -> w572
          event Timeout {
            n301 = event-data() -> ()  [unwired: 1 in, 2 out]
          }
          event "Down Button": Mouse Down {
            w934 = 0
            n302 = event-data() -> ()  [unwired: 1 in, 7 out]
            n303 = local read "Data File"() -> (w950:path)
            n304 = call "Recorded Values.vi"("Path"=w950) -> ("Recorded Char"=w952:T5, "Recorded Prop"=w953:T6, "Fabrication Prop"=w951:T7)  [unwired: 8 in]
            n305 = Unbundle By Name(w952) -> ("Mobility-Sat"=w966:dbl, "Moblitity-Lin"=w967:dbl, "On/Off"=w968:dbl, "Threshold Voltage"=w969:dbl, "STS"=w970:dbl, "Trap Density-VT"=w971:dbl, "Trap Density-STS"=w972:dbl)  [unwired: 1 out]
            n306 = Unbundle By Name(w951) -> ("Date Created"=w973:string, "Material"=w954:string, "Solvent"=w955:string, "Concentration"=w956:dbl, "Method"=w957:string, "Dielectric (nm)"=w958:dbl, "Treatment"=w959:string, "Comments"=w960:string)
            n307 = Unbundle By Name(w953) -> ("Date Recorded"=w961:string, "Index"=w962:string, "Length"=w963:dbl, "Width"=w964:dbl, "Sample Temp"=w965:dbl)
            n308 = local write "Date Created"(w973) -> ()
            n309 = local write "Rec: VT-Sat"(w969) -> ()
            n310 = local write "Rec: Material"(w954) -> ()
            n311 = local write "Rec: Concentration"(w956) -> ()
            n312 = local write "Rec: Method"(w957) -> ()
            n313 = local write "Rec: Dielectric (d)"(w958) -> ()
            n314 = local write "Surface Treatment:"(w959) -> ()
            n315 = local write "Comments"(w960) -> ()
            n316 = local write "Index"(w962) -> ()
            n317 = local write "Rec: Mobility-Sat"(w966) -> ()
            n318 = local write "Rec: Mobility-Lin"(w967) -> ()
            n319 = local write "Rec: On/Off"(w968) -> ()
            n320 = local write "Rec: STS"(w970) -> ()
            n321 = local write "Rec: Trap Density-VT"(w971) -> ()
            n322 = local write "Rec: Trap Density-STS"(w972) -> ()
            n323 = local write "Rec: Solvent"(w955) -> ()
            n324 = local write "Date Recorded"(w961) -> ()
            n325 = local write "Rec: Length"(w963) -> ()
            n326 = local write "Rec: Width"(w964) -> ()
            n327 = local write "Rec: Temp"(w965) -> ()
            n328 = local read "Data File"() -> (w939:path)
            n329 = Strip Path(path=w939) -> (stripped path=w930:path, name=w948:string)
            n330 = local write "Data Folder"(w930) -> ()
            n331 = List Folder(path=w930) -> (filenames=w944:string[], error out=w884:errorcluster)  [unwired: 3 in, 2 out]
            n332 = local read "Folder Index"() -> (w886:dbl)
            n333 = property on="Image Out" class="ImageControl"() -> (error out=w887:errorcluster, "Image Center Position"=w891:cluster{"X":u32, "Y":u32})  [unwired: 2 in, 1 out]
            n334 = Array Size(array=w944) -> (size(s)=w940:i32)
            n335 = Search 1D Array(1D array=w944, element=w948) -> (index of element=w941:i32)  [unwired: 1 in]
            n336 = Decrement(x=w940) -> (x-1=w942:i32)
            n337 = Equal?(x=w941, y=w942) -> (x = y?=w943:bool)
            n338 = invoke on="Image Out" class="ImageControl" method="Clear ROI"() -> ()  [unwired: 3 in, 3 out]
            n339 = case shown="False" w943 {
              tunnel: w886 -> [w1101 _]
              tunnel: [w1100 0] -> w885
              tunnel: w884 -> [w1099 w1102]
              tunnel: [w1099 w1102] -> w883
              frame False {
                n340 = Increment(x=w1101) -> (x+1=w1100:dbl)
              }
              frame True {
              }
            }
            n341 = Unbundle(w891) -> ("X"=w889:u32)  [unwired: 1 out]
            n342 = local write "Folder Index"(w885) -> ()
            n343 = Bundle("X"=w889, 0) -> (w890:cluster{"X":u32, i32})  [unwired: 1 in]
            n344 = property on="Image Out" class="ImageControl"(error in=w887, "Image Center Position"=w890) -> ()  [unwired: 1 in, 2 out]
            n345 = Path To String(path=w930) -> (string=w949:string)
            n346 = Index Array(array=w944, index=w885) -> (element=w945:string)
            n347 = local write "Data Name:"(w945) -> ()
            n348 = Concatenate Strings(w949, "\\", w945) -> (w947:string)
            n349 = String To Path(string=w947) -> (path=w882:path)
            n350 = local read "NumPts 2"() -> (w877:dbl)
            n351 = local read "NumPts"() -> (w881:dbl)
            n352 = local write "Data File"(w882) -> ()
            n353 = call-poly <vilib>:"Read From Spreadsheet File.vi"("file path (dialog if empty)"=w882) -> ("all rows"=w936:string[][])  [unwired: 6 in, 4 out]
            n354 = call "Mobility-Vt Calculator-File.vi"("NumPts"=w881, "Path"=w882) -> ("XY Graph-Sat"=w879:cluster{dbl[], dbl[]}[], "XY Graph-Lin"=w865:cluster{dbl[], dbl[]}[], "Output"=w880:T8, "Index-Sat"=w878:dbl, "Index-Lin"=w863:dbl)  [unwired: 4 in, 1 out]
            n355 = local read "New: Dielectric"() -> (w860:dbl)
            n356 = call "STS Calculator-File.vi"("NumPts"=w877, "Path"=w882) -> ("STS Index-Sat"=w876:dbl, "XY Graph-Sat"=w875:cluster{dbl[], dbl[]}[], "Ouput"=w874:cluster{"STS-Sat":dbl, "STS-Lin":dbl})  [unwired: 5 in, 2 out]
            n357 = local read "New: Temp"() -> (w857:dbl)
            n358 = Unbundle By Name(w880) -> ("Mobility-Sat"=w873:dbl, "Vt-Sat"=w859:dbl, "Mobility-Lin"=w872:dbl, "Vt-Lin"=w871:dbl)
            n359 = Unbundle By Name(w874) -> ("STS-Sat"=w858:dbl)  [unwired: 1 out]
            n360 = local write "Index 2"(w876) -> ()
            n361 = local write "XY Graph 2"(w875) -> ()
            n362 = local write "MobVi Index"(w878) -> ()
            n363 = local write "Slide"(w878) -> ()
            n364 = local write "XY Graph"(w879) -> ()
            n365 = Array Size(array=w936) -> (size(s)=w935:i32[])
            n366 = call "Trap Density_VT.vi"("VT"=w859, "Dielectric"=w860) -> ("Trap Density-VT"=w856:dbl)
            n367 = call "Trap Density_STS.vi"("Temp (T) [K]"=w857, "S.T.S. (S)"=w858, "Dielectric"=w860) -> ("Trap Density (N)"=w855:dbl)  [unwired: 8 in]
            n368 = local write "Calc: Mobility-Sat"(w873) -> ()
            n369 = local write "Calc: STS"(w858) -> ()
            n370 = local write "Calc: Mobility-Lin"(w871) -> ()
            n371 = local write "Calc: VT-Sat"(w859) -> ()
            n372 = local write "Calc: VT-Lin"(w872) -> ()
            n373 = local write "Calc: Trap Density-VT"(w856) -> ()
            n374 = local write "Calc: Trap Density-STS"(w855) -> ()
            n375 = local write "New: Trap Density-STS"(w855) -> ()
            n376 = local write "New: Trap Density-VT"(w856) -> ()
            n377 = Index Array(array=w935, index=w934) -> (element=w916:i32)
            n378 = Decimate 1D Array(w875) -> (w910:cluster{dbl[], dbl[]}[])  [unwired: 1 out]
            n379 = Decimate 1D Array(w879) -> (w920:cluster{dbl[], dbl[]}[])  [unwired: 1 out]
            n380 = Decimate 1D Array(w865) -> (w870:cluster{dbl[], dbl[]}[])  [unwired: 1 out]
            n381 = Array Subset(array=w936, index (row)=w934, index (col)=w934, length (col)=3) -> (w937:string[][])  [unwired: 1 in]
            n382 = Array To Cluster(array=w910) -> (cluster=w908:T9)
            n383 = Array To Cluster(array=w920) -> (cluster=w922:T9)
            n384 = Reshape Array(w937, w916) -> (w923:string[])
            n385 = Array To Cluster(array=w870) -> (cluster=w869:T9)
            n386 = Subtract(x=w916, y=20) -> (x-y=w915:i32)
            n387 = local write "New: Mobility-Sat"(w873) -> ()
            n388 = local write "New: Mobility-Lin"(w872) -> ()
            n389 = local write "New: VT-Sat"(w859) -> ()
            n390 = local write "New: VT-Lin"(w871) -> ()
            n391 = property on="Slide" class="Slide (strict)"("Scale.Maximum"=w915) -> ()  [unwired: 2 in, 2 out]
            n392 = Unbundle(w908) -> ("[0]"=w909:cluster{dbl[], dbl[]})  [unwired: 8 out]
            n393 = Unbundle(w922) -> ("[0]"=w921:cluster{dbl[], dbl[]})  [unwired: 8 out]
            n394 = Unbundle(w869) -> ("[0]"=w866:cluster{dbl[], dbl[]})  [unwired: 8 out]
            n395 = Search 1D Array(1D array=w923, element="Index:") -> (index of element=w931:i32)  [unwired: 1 in]
            n396 = local read "NumPts"() -> (w864:dbl)
            n397 = Unbundle(w866) -> (w868:dbl[], w867:dbl[])
            n398 = Increment(x=w931) -> (x+1=w932:i32)
            n399 = Unbundle(w909) -> (w907:dbl[], w906:dbl[])
            n400 = Unbundle(w921) -> (w912:dbl[], w911:dbl[])
            n401 = Array Subset(array=w868, index=w863, length=w864) -> (w862:dbl[])
            n402 = Array Subset(array=w867, index=w863, length=w864) -> (w861:dbl[])
            n403 = Array Subset(array=w907, index=w876, length=w877) -> (w914:dbl[])
            n404 = Array Subset(array=w906, index=w876, length=w877) -> (w913:dbl[])
            n405 = Array Subset(array=w912, index=w878, length=w881) -> (w919:dbl[])
            n406 = Array Subset(array=w911, index=w878, length=w881) -> (w918:dbl[])
            n407 = Index Array(array=w923, index=w932) -> (element=w895:string)
            n408 = local write "Lin-Vg Array-Used"(w862) -> ()
            n409 = local write "Sat Vg Array-Used"(w919) -> ()
            n410 = local write "Vg Array-Log-Used"(w913) -> ()
            n411 = local write "Lin Id-Used"(w861) -> ()
            n412 = local read "Image Folder"() -> (w893:path)
            n413 = local write "Sat Id-Used"(w918) -> ()
            n414 = local write "Sat Id-Log-Used"(w914) -> ()
            n415 = List Folder(path=w893, error in=w883) -> (filenames=w929:string[], error out=w896:errorcluster)  [unwired: 2 in, 2 out]
            n416 = while {
              tunnel: w929 -> [w986]
              tunnel: w895 -> [w984]
              tunnel: [w983] -> _
              tunnel: [w983] -> w928
              tunnel: w916 -> [w982]
              i -> [w983]
              stop <- w979 stop-if-true
              n417 = Index Array(array=w986, index=w983) -> (element=w987:string)
              n418 = xnode "Match Regular Expression"("input string"=w987, "regular expression"=w984) -> ("whole match"=w985:string)  [unwired: 4 in, 4 out]
              n419 = Equal?(x=w985, y=w984) -> (x = y?=w981:bool)
              n420 = Equal?(x=w982, y=w983) -> (x = y?=w980:bool)
              n421 = Or(x=w981, y=w980) -> (x .or. y?=w979:bool)
            }
            n422 = Build Path(base path=w893, name or relative path="ROI") -> (appended path=w892:path)
            n423 = Path To String(path=w893) -> (string=w926:string)
            n424 = Index Array(array=w929, index=w928) -> (element=w904:string)
            n425 = invoke on="Image Out" class="ImageControl" method="Clear ROI"(error in=w896) -> (error out=w899:errorcluster)  [unwired: 2 in, 2 out]
            n426 = local write "Image Name"(w904) -> ()
            n427 = Build Path(base path=w892, name or relative path=w895) -> (appended path=w900:path)
            n428 = call <vilib>:"Check if File or Folder Exists.vi"("error in (no error)"=w899, "path"=w900) -> ("file or folder exists?"=w897:bool, "dup path"=w898:path)  [unwired: 7 in, 1 out]
            n429 = Concatenate Strings(w926, "\\", w904) -> (w925:string)
            n430 = case shown="True" w897 {
              tunnel: w898 -> [_ w974]
              frame False {
              }
              frame True {
                n431 = Read from Text File(file (use dialog)=w974) -> (text=w978:string)  [unwired: 3 in, 3 out]
                n432 = property on="Image Out" class="ImageControl"() -> ("ROI"=w975:T10)  [unwired: 2 in, 2 out]
                n433 = Unflatten From String(type=w975, binary string=w978) -> (value=w976:T10, error out=w977:errorcluster)  [unwired: 3 in, 1 out]
                n434 = property on="Image Out" class="ImageControl"(error in=w977, "ROI"=w976) -> ()  [unwired: 1 in, 2 out]
              }
            }
            n435 = String To Path(string=w925) -> (path=w903:path)
            n436 = Empty String/Path?(string/path=w904) -> (empty?=w905:bool)
            n437 = local read "No Image"() -> (w901:path)
            n438 = Select(t=w901, s=w905, f=w903) -> (s? t:f=w902:path)
            n439 = local write "Image File"(w902) -> ()
            n440 = call "Vision Acquisition4"("Image Path"=w902) -> ("Image Out"=w927:T2)  [unwired: 25 in, 1 out]
            n441 = local write "Image Out"(w927) -> ()
            n442 = local write "Image Out 2"(w927) -> ()
          }
          event "Data File": Value Change {
            w1207 = 0
            n443 = event-data() -> ()  [unwired: 1 in, 5 out]
            n444 = local read "Data File"() -> (w1156:path)
            n445 = call "Recorded Values.vi"("Path"=w1156) -> ("Recorded Char"=w1154:T5, "Recorded Prop"=w1153:T6, "Fabrication Prop"=w1155:T7)  [unwired: 8 in]
            n446 = Unbundle By Name(w1154) -> ("Mobility-Sat"=w1140:dbl, "Moblitity-Lin"=w1139:dbl, "On/Off"=w1138:dbl, "Threshold Voltage"=w1137:dbl, "STS"=w1136:dbl, "Trap Density-VT"=w1135:dbl, "Trap Density-STS"=w1134:dbl)  [unwired: 1 out]
            n447 = Unbundle By Name(w1155) -> ("Date Created"=w1133:string, "Material"=w1152:string, "Solvent"=w1151:string, "Concentration"=w1150:dbl, "Method"=w1149:string, "Dielectric (nm)"=w1148:dbl, "Treatment"=w1147:string, "Comments"=w1146:string)
            n448 = Unbundle By Name(w1153) -> ("Date Recorded"=w1145:string, "Index"=w1144:string, "Length"=w1143:dbl, "Width"=w1142:dbl, "Sample Temp"=w1141:dbl)
            n449 = local write "Date Created"(w1133) -> ()
            n450 = local read "Data File"() -> (w1203:path)
            n451 = local write "Rec: Material"(w1152) -> ()
            n452 = local write "Rec: VT-Sat"(w1137) -> ()
            n453 = local write "Rec: Concentration"(w1150) -> ()
            n454 = local write "Rec: Method"(w1149) -> ()
            n455 = local write "Rec: Dielectric (d)"(w1148) -> ()
            n456 = local write "Surface Treatment:"(w1147) -> ()
            n457 = local write "Comments"(w1146) -> ()
            n458 = local write "Index"(w1144) -> ()
            n459 = local write "Rec: Mobility-Sat"(w1140) -> ()
            n460 = local write "Rec: Mobility-Lin"(w1139) -> ()
            n461 = local write "Rec: On/Off"(w1138) -> ()
            n462 = local write "Rec: STS"(w1136) -> ()
            n463 = local write "Rec: Trap Density-VT"(w1135) -> ()
            n464 = local write "Rec: Trap Density-STS"(w1134) -> ()
            n465 = Strip Path(path=w1203) -> (stripped path=w1202:path, name=w1216:string)
            n466 = local write "Rec: Solvent"(w1151) -> ()
            n467 = local write "Date Recorded"(w1145) -> ()
            n468 = local write "Rec: Length"(w1143) -> ()
            n469 = local write "Rec: Width"(w1142) -> ()
            n470 = local write "Rec: Temp"(w1141) -> ()
            n471 = local write "Data Folder"(w1202) -> ()
            n472 = property on="Image Out" class="ImageControl"() -> (error out=w1158:errorcluster, "Image Center Position"=w1162:cluster{"X":u32, "Y":u32})  [unwired: 2 in, 1 out]
            n473 = List Folder(path=w1202) -> (filenames=w1212:string[], error out=w1168:errorcluster)  [unwired: 3 in, 2 out]
            n474 = Search 1D Array(1D array=w1212, element=w1216) -> (index of element=w1157:i32)  [unwired: 1 in]
            n475 = local write "Folder Index"(w1157) -> ()
            n476 = Unbundle(w1162) -> ("X"=w1160:u32)  [unwired: 1 out]
            n477 = Path To String(path=w1202) -> (string=w1217:string)
            n478 = Index Array(array=w1212, index=w1157) -> (element=w1213:string)
            n479 = Bundle("X"=w1160, 0) -> (w1161:cluster{"X":u32, i32})  [unwired: 1 in]
            n480 = local write "Data Name:"(w1213) -> ()
            n481 = property on="Image Out" class="ImageControl"(error in=w1158, "Image Center Position"=w1161) -> ()  [unwired: 1 in, 2 out]
            n482 = Concatenate Strings(w1217, "\\", w1213) -> (w1215:string)
            n483 = String To Path(string=w1215) -> (path=w1132:path)
            n484 = local read "NumPts 2"() -> (w1127:dbl)
            n485 = local write "Data File"(w1132) -> ()
            n486 = local read "NumPts"() -> (w1128:dbl)
            n487 = local read "New: Dielectric"() -> (w1109:dbl)
            n488 = local read "New: Temp"() -> (w1108:dbl)
            n489 = call-poly <vilib>:"Read From Spreadsheet File.vi"("file path (dialog if empty)"=w1132) -> ("all rows"=w1209:string[][])  [unwired: 6 in, 4 out]
            n490 = call "STS Calculator-File.vi"("NumPts"=w1127, "Path"=w1132) -> ("STS Index-Sat"=w1125:dbl, "XY Graph-Sat"=w1126:cluster{dbl[], dbl[]}[], "Ouput"=w1124:cluster{"STS-Sat":dbl, "STS-Lin":dbl})  [unwired: 5 in, 2 out]
            n491 = call "Mobility-Vt Calculator-File.vi"("NumPts"=w1128, "Path"=w1132) -> ("XY Graph-Sat"=w1131:cluster{dbl[], dbl[]}[], "XY Graph-Lin"=w1121:cluster{dbl[], dbl[]}[], "Output"=w1129:T8, "Index-Sat"=w1130:dbl, "Index-Lin"=w1116:dbl)  [unwired: 4 in, 1 out]
            n492 = Unbundle By Name(w1129) -> ("Mobility-Sat"=w1112:dbl, "Vt-Sat"=w1104:dbl, "Mobility-Lin"=w1111:dbl, "Mobility-Lin"=w1110:dbl)
            n493 = local write "Index 2"(w1125) -> ()
            n494 = local write "XY Graph 2"(w1126) -> ()
            n495 = Unbundle By Name(w1124) -> ("STS-Sat"=w1105:dbl)  [unwired: 1 out]
            n496 = local write "MobVi Index"(w1130) -> ()
            n497 = Array Size(array=w1209) -> (size(s)=w1208:i32[])
            n498 = call "Trap Density_VT.vi"("VT"=w1104, "Dielectric"=w1109) -> ("Trap Density-VT"=w1107:dbl)
            n499 = call "Trap Density_STS.vi"("Temp (T) [K]"=w1108, "S.T.S. (S)"=w1105, "Dielectric"=w1109) -> ("Trap Density (N)"=w1106:dbl)  [unwired: 8 in]
            n500 = local write "Slide"(w1130) -> ()
            n501 = local write "Calc: Mobility-Sat"(w1112) -> ()
            n502 = local write "Calc: Mobility-Lin"(w1110) -> ()
            n503 = local write "Calc: VT-Sat"(w1104) -> ()
            n504 = local write "Calc: VT-Lin"(w1111) -> ()
            n505 = local write "Calc: STS"(w1105) -> ()
            n506 = local write "Calc: Trap Density-VT"(w1107) -> ()
            n507 = local write "Calc: Trap Density-STS"(w1106) -> ()
            n508 = local write "New: Trap Density-STS"(w1106) -> ()
            n509 = local write "New: Trap Density-VT"(w1107) -> ()
            n510 = Decimate 1D Array(w1121) -> (w1123:cluster{dbl[], dbl[]}[])  [unwired: 1 out]
            n511 = Decimate 1D Array(w1126) -> (w1183:cluster{dbl[], dbl[]}[])  [unwired: 1 out]
            n512 = Index Array(array=w1208, index=w1207) -> (element=w1189:i32)
            n513 = Decimate 1D Array(w1131) -> (w1192:cluster{dbl[], dbl[]}[])  [unwired: 1 out]
            n514 = local write "XY Graph"(w1131) -> ()
            n515 = Array Subset(array=w1209, index (row)=w1207, index (col)=w1207, length (col)=3) -> (w1210:string[][])  [unwired: 1 in]
            n516 = Array To Cluster(array=w1123) -> (cluster=w1122:T9)
            n517 = local write "New: STS"(w1105) -> ()
            n518 = Array To Cluster(array=w1183) -> (cluster=w1181:T9)
            n519 = Array To Cluster(array=w1192) -> (cluster=w1194:T9)
            n520 = Reshape Array(w1210, w1189) -> (w1195:string[])
            n521 = local write "New: Mobility-Sat"(w1112) -> ()
            n522 = local write "New: Mobility-Lin"(w1111) -> ()
            n523 = Subtract(x=w1189, y=20) -> (x-y=w1187:i32)
            n524 = local write "New: VT-Sat"(w1104) -> ()
            n525 = local write "New: VT-Lin"(w1110) -> ()
            n526 = Unbundle(w1122) -> ("[0]"=w1120:cluster{dbl[], dbl[]})  [unwired: 8 out]
            n527 = property on="Slide" class="Slide (strict)"("Scale.Maximum"=w1187) -> ()  [unwired: 2 in, 2 out]
            n528 = local read "NumPts"() -> (w1117:dbl)
            n529 = Unbundle(w1120) -> (w1119:dbl[], w1118:dbl[])
            n530 = Unbundle(w1181) -> ("[0]"=w1182:cluster{dbl[], dbl[]})  [unwired: 8 out]
            n531 = Unbundle(w1194) -> ("[0]"=w1193:cluster{dbl[], dbl[]})  [unwired: 8 out]
            n532 = Search 1D Array(1D array=w1195, element="Index:") -> (index of element=w1204:i32)  [unwired: 1 in]
            n533 = local read "NumPts"() -> (w1113:dbl)
            n534 = Array Subset(array=w1119, index=w1116, length=w1117) -> (w1115:dbl[])
            n535 = Array Subset(array=w1118, index=w1116, length=w1117) -> (w1114:dbl[])
            n536 = Increment(x=w1204) -> (x+1=w1205:i32)
            n537 = Unbundle(w1182) -> (w1179:dbl[], w1178:dbl[])
            n538 = Unbundle(w1193) -> (w1180:dbl[], w1184:dbl[])
            n539 = local read "Image Folder"() -> (w1164:path)
            n540 = local write "Lin-Vg Array-Used"(w1115) -> ()
            n541 = Array Subset(array=w1179, index=w1125, length=w1127) -> (w1186:dbl[])
            n542 = Array Subset(array=w1178, index=w1125, length=w1127) -> (w1185:dbl[])
            n543 = Array Subset(array=w1180, index=w1130, length=w1113) -> (w1191:dbl[])
            n544 = Array Subset(array=w1184, index=w1130, length=w1113) -> (w1190:dbl[])
            n545 = Index Array(array=w1195, index=w1205) -> (element=w1166:string)
            n546 = local write "Lin Id-Used"(w1114) -> ()
            n547 = local write "Sat Vg Array-Used"(w1191) -> ()
            n548 = local write "Vg Array-Log-Used"(w1185) -> ()
            n549 = local write "Sat Id-Log-Used"(w1186) -> ()
            n550 = local write "Sat Id-Used"(w1190) -> ()
            n551 = local write "Index"(w1166) -> ()
            n552 = List Folder(path=w1164, error in=w1168) -> (filenames=w1200:string[], error out=w1167:errorcluster)  [unwired: 2 in, 2 out]
            n553 = Build Path(base path=w1164, name or relative path="ROI") -> (appended path=w1163:path)
            n554 = while {
              tunnel: w1200 -> [w1230]
              tunnel: w1166 -> [w1228]
              tunnel: [w1227] -> _
              tunnel: [w1227] -> w1199
              tunnel: w1189 -> [w1226]
              i -> [w1227]
              stop <- w1223 stop-if-true
              n555 = Index Array(array=w1230, index=w1227) -> (element=w1231:string)
              n556 = xnode "Match Regular Expression"("input string"=w1231, "regular expression"=w1228) -> ("whole match"=w1229:string)  [unwired: 4 in, 4 out]
              n557 = Equal?(x=w1229, y=w1228) -> (x = y?=w1225:bool)
              n558 = Equal?(x=w1226, y=w1227) -> (x = y?=w1224:bool)
              n559 = Or(x=w1225, y=w1224) -> (x .or. y?=w1223:bool)
            }
            n560 = invoke on="Image Out" class="ImageControl" method="Clear ROI"(error in=w1167) -> (error out=w1171:errorcluster)  [unwired: 2 in, 2 out]
            n561 = Build Path(base path=w1163, name or relative path=w1166) -> (appended path=w1172:path)
            n562 = call <vilib>:"Check if File or Folder Exists.vi"("error in (no error)"=w1171, "path"=w1172) -> ("file or folder exists?"=w1169:bool, "dup path"=w1170:path)  [unwired: 7 in, 1 out]
            n563 = case shown="True" w1169 {
              tunnel: w1170 -> [_ w1218]
              frame False {
              }
              frame True {
                n564 = Read from Text File(file (use dialog)=w1218) -> (text=w1222:string)  [unwired: 3 in, 3 out]
                n565 = property on="Image Out" class="ImageControl"() -> ("ROI"=w1219:T10)  [unwired: 2 in, 2 out]
                n566 = Unflatten From String(type=w1219, binary string=w1222) -> (value=w1220:T10, error out=w1221:errorcluster)  [unwired: 3 in, 1 out]
                n567 = property on="Image Out" class="ImageControl"(error in=w1221, "ROI"=w1220) -> ()  [unwired: 1 in, 2 out]
              }
            }
            n568 = invoke on="Image Out" class="ImageControl" method="Clear ROI"() -> ()  [unwired: 3 in, 3 out]
            n569 = Path To String(path=w1164) -> (string=w1198:string)
            n570 = Index Array(array=w1200, index=w1199) -> (element=w1176:string)
            n571 = Concatenate Strings(w1198, "\\", w1176) -> (w1197:string)
            n572 = local write "Image Name"(w1176) -> ()
            n573 = String To Path(string=w1197) -> (path=w1175:path)
            n574 = Empty String/Path?(string/path=w1176) -> (empty?=w1177:bool)
            n575 = local read "No Image"() -> (w1173:path)
            n576 = Select(t=w1173, s=w1177, f=w1175) -> (s? t:f=w1174:path)
            n577 = local write "Image File"(w1174) -> ()
            n578 = call "Vision Acquisition3"("Image Path"=w1174) -> ("Image Out"=w1201:T2)  [unwired: 25 in, 1 out]
            n579 = local write "Image Out"(w1201) -> ()
            n580 = local write "Image Out 2"(w1201) -> ()
          }
          event "Up Button": Mouse Down {
            w1447 = 0
            n581 = event-data() -> ()  [unwired: 1 in, 5 out]
            n582 = local read "Data File"() -> (w1394:path)
            n583 = call "Recorded Values.vi"("Path"=w1394) -> ("Recorded Char"=w1392:T5, "Recorded Prop"=w1391:T6, "Fabrication Prop"=w1393:T7)  [unwired: 8 in]
            n584 = Unbundle By Name(w1392) -> ("Mobility-Sat"=w1378:dbl, "Moblitity-Lin"=w1377:dbl, "On/Off"=w1376:dbl, "Threshold Voltage"=w1375:dbl, "STS"=w1374:dbl, "Trap Density-VT"=w1373:dbl, "Trap Density-STS"=w1372:dbl)  [unwired: 1 out]
            n585 = Unbundle By Name(w1393) -> ("Date Created"=w1371:string, "Material"=w1390:string, "Solvent"=w1389:string, "Concentration"=w1388:dbl, "Method"=w1387:string, "Dielectric (nm)"=w1386:dbl, "Treatment"=w1385:string, "Comments"=w1384:string)
            n586 = Unbundle By Name(w1391) -> ("Date Recorded"=w1383:string, "Index"=w1382:string, "Length"=w1381:dbl, "Width"=w1380:dbl, "Sample Temp"=w1379:dbl)
            n587 = local write "Date Created"(w1371) -> ()
            n588 = local write "Rec: Material"(w1390) -> ()
            n589 = local write "Rec: VT-Sat"(w1375) -> ()
            n590 = local write "Rec: Solvent"(w1389) -> ()
            n591 = local write "Rec: Concentration"(w1388) -> ()
            n592 = local write "Rec: Method"(w1387) -> ()
            n593 = local write "Rec: Dielectric (d)"(w1386) -> ()
            n594 = local write "Surface Treatment:"(w1385) -> ()
            n595 = local write "Comments"(w1384) -> ()
            n596 = local write "Index"(w1382) -> ()
            n597 = local write "Rec: Mobility-Sat"(w1378) -> ()
            n598 = local write "Rec: Mobility-Lin"(w1377) -> ()
            n599 = local write "Rec: On/Off"(w1376) -> ()
            n600 = local write "Rec: STS"(w1374) -> ()
            n601 = local write "Rec: Trap Density-VT"(w1373) -> ()
            n602 = local write "Rec: Trap Density-STS"(w1372) -> ()
            n603 = local write "Date Recorded"(w1383) -> ()
            n604 = local write "Rec: Length"(w1381) -> ()
            n605 = local write "Rec: Width"(w1380) -> ()
            n606 = local write "Rec: Temp"(w1379) -> ()
            n607 = local read "Data File"() -> (w1443:path)
            n608 = Strip Path(path=w1443) -> (stripped path=w1442:path, name=w1458:string)
            n609 = local write "Data Folder"(w1442) -> ()
            n610 = List Folder(path=w1442) -> (filenames=w1452:string[], error out=w1409:errorcluster)  [unwired: 3 in, 2 out]
            n611 = Array Size(array=w1452) -> (size(s)=w1397:i32)
            n612 = Search 1D Array(1D array=w1452, element=w1458) -> (index of element=w1453:i32)  [unwired: 1 in]
            n613 = Equal To 0?(x=w1453) -> (x = 0?=w1454:bool)
            n614 = local read "Folder Index"() -> (w1396:dbl)
            n615 = property on="Image Out" class="ImageControl"() -> (error out=w1399:errorcluster, "Image Center Position"=w1403:cluster{"X":u32, "Y":u32})  [unwired: 2 in, 1 out]
            n616 = case shown="True" w1454 {
              tunnel: w1396 -> [w1586 _]
              tunnel: [w1585 w1587] -> w1395
              tunnel: w1397 -> [_ w1588]
              frame False {
                n617 = Decrement(x=w1586) -> (x-1=w1585:dbl)
              }
              frame True {
                n618 = Decrement(x=w1588) -> (x-1=w1587:i32)
              }
            }
            n619 = local write "Folder Index"(w1395) -> ()
            n620 = Unbundle(w1403) -> ("X"=w1401:u32)  [unwired: 1 out]
            n621 = Bundle("X"=w1401, 0) -> (w1402:cluster{"X":u32, i32})  [unwired: 1 in]
            n622 = Path To String(path=w1442) -> (string=w1459:string)
            n623 = Index Array(array=w1452, index=w1395) -> (element=w1455:string)
            n624 = local write "Data Name:"(w1455) -> ()
            n625 = property on="Image Out" class="ImageControl"(error in=w1399, "Image Center Position"=w1402) -> ()  [unwired: 1 in, 2 out]
            n626 = Concatenate Strings(w1459, "\\", w1455) -> (w1457:string)
            n627 = String To Path(string=w1457) -> (path=w1370:path)
            n628 = local read "NumPts 2"() -> (w1365:dbl)
            n629 = local write "Data File"(w1370) -> ()
            n630 = local read "NumPts"() -> (w1369:dbl)
            n631 = local read "New: Dielectric"() -> (w1348:dbl)
            n632 = call "Mobility-Vt Calculator-File.vi"("NumPts"=w1369, "Path"=w1370) -> ("XY Graph-Sat"=w1367:cluster{dbl[], dbl[]}[], "XY Graph-Lin"=w1352:cluster{dbl[], dbl[]}[], "Output"=w1368:T8, "Index-Sat"=w1366:dbl, "Index-Lin"=w1353:dbl)  [unwired: 4 in, 1 out]
            n633 = call "STS Calculator-File.vi"("NumPts"=w1365, "Path"=w1370) -> ("STS Index-Sat"=w1364:dbl, "XY Graph-Sat"=w1363:cluster{dbl[], dbl[]}[], "Ouput"=w1362:cluster{"STS-Sat":dbl, "STS-Lin":dbl})  [unwired: 5 in, 2 out]
            n634 = call-poly <vilib>:"Read From Spreadsheet File.vi"("file path (dialog if empty)"=w1370) -> ("all rows"=w1449:string[][])  [unwired: 6 in, 4 out]
            n635 = local read "New: Temp"() -> (w1347:dbl)
            n636 = Unbundle By Name(w1368) -> ("Mobility-Sat"=w1351:dbl, "Vt-Sat"=w1343:dbl, "Mobility-Lin"=w1350:dbl, "Mobility-Lin"=w1349:dbl)
            n637 = Unbundle By Name(w1362) -> ("STS-Sat"=w1344:dbl)  [unwired: 1 out]
            n638 = local write "Index 2"(w1364) -> ()
            n639 = local write "XY Graph 2"(w1363) -> ()
            n640 = local write "MobVi Index"(w1366) -> ()
            n641 = local write "Slide"(w1366) -> ()
            n642 = local write "XY Graph"(w1367) -> ()
            n643 = Array Size(array=w1449) -> (size(s)=w1448:i32[])
            n644 = local write "Calc: Mobility-Sat"(w1351) -> ()
            n645 = local write "Calc: Mobility-Lin"(w1349) -> ()
            n646 = call "Trap Density_VT.vi"("VT"=w1343, "Dielectric"=w1348) -> ("Trap Density-VT"=w1346:dbl)
            n647 = call "Trap Density_STS.vi"("Temp (T) [K]"=w1347, "S.T.S. (S)"=w1344, "Dielectric"=w1348) -> ("Trap Density (N)"=w1345:dbl)  [unwired: 8 in]
            n648 = local write "Calc: VT-Sat"(w1343) -> ()
            n649 = local write "Calc: VT-Lin"(w1350) -> ()
            n650 = local write "Calc: STS"(w1344) -> ()
            n651 = local write "New: STS"(w1344) -> ()
            n652 = Decimate 1D Array(w1352) -> (w1361:cluster{dbl[], dbl[]}[])  [unwired: 1 out]
            n653 = local write "Calc: Trap Density-VT"(w1346) -> ()
            n654 = local write "Calc: Trap Density-STS"(w1345) -> ()
            n655 = local write "New: Trap Density-STS"(w1345) -> ()
            n656 = local write "New: Trap Density-VT"(w1346) -> ()
            n657 = Decimate 1D Array(w1363) -> (w1426:cluster{dbl[], dbl[]}[])  [unwired: 1 out]
            n658 = Index Array(array=w1448, index=w1447) -> (element=w1432:i32)
            n659 = Decimate 1D Array(w1367) -> (w1436:cluster{dbl[], dbl[]}[])  [unwired: 1 out]
            n660 = Array To Cluster(array=w1361) -> (cluster=w1360:T9)
            n661 = Array Subset(array=w1449, index (row)=w1447, index (col)=w1447, length (col)=3) -> (w1450:string[][])  [unwired: 1 in]
            n662 = local write "New: Mobility-Sat"(w1351) -> ()
            n663 = local write "New: Mobility-Lin"(w1350) -> ()
            n664 = Array To Cluster(array=w1426) -> (cluster=w1424:T9)
            n665 = Array To Cluster(array=w1436) -> (cluster=w1438:T9)
            n666 = Reshape Array(w1450, w1432) -> (w1439:string[])
            n667 = local write "New: VT-Sat"(w1343) -> ()
            n668 = local write "New: VT-Lin"(w1349) -> ()
            n669 = Subtract(x=w1432, y=20) -> (x-y=w1431:i32)
            n670 = Unbundle(w1360) -> ("[0]"=w1357:cluster{dbl[], dbl[]})  [unwired: 8 out]
            n671 = property on="Slide" class="Slide (strict)"("Scale.Maximum"=w1431) -> ()  [unwired: 2 in, 2 out]
            n672 = Unbundle(w1424) -> ("[0]"=w1425:cluster{dbl[], dbl[]})  [unwired: 8 out]
            n673 = Unbundle(w1438) -> ("[0]"=w1437:cluster{dbl[], dbl[]})  [unwired: 8 out]
            n674 = local read "NumPts"() -> (w1354:dbl)
            n675 = Unbundle(w1357) -> (w1356:dbl[], w1355:dbl[])
            n676 = Search 1D Array(1D array=w1439, element="Index:") -> (index of element=w1444:i32)  [unwired: 1 in]
            n677 = Increment(x=w1444) -> (x+1=w1445:i32)
            n678 = Unbundle(w1425) -> (w1423:dbl[], w1422:dbl[])
            n679 = Unbundle(w1437) -> (w1430:dbl[], w1429:dbl[])
            n680 = Array Subset(array=w1356, index=w1353, length=w1354) -> (w1358:dbl[])
            n681 = Array Subset(array=w1355, index=w1353, length=w1354) -> (w1359:dbl[])
            n682 = local read "Image Folder"() -> (w1398:path)
            n683 = local write "Lin-Vg Array-Used"(w1358) -> ()
            n684 = Array Subset(array=w1423, index=w1364, length=w1365) -> (w1428:dbl[])
            n685 = Array Subset(array=w1422, index=w1364, length=w1365) -> (w1427:dbl[])
            n686 = Array Subset(array=w1430, index=w1366, length=w1369) -> (w1435:dbl[])
            n687 = Array Subset(array=w1429, index=w1366, length=w1369) -> (w1434:dbl[])
            n688 = local write "Lin Id-Used"(w1359) -> ()
            n689 = Index Array(array=w1439, index=w1445) -> (element=w1405:string)
            n690 = local write "Sat Vg Array-Used"(w1435) -> ()
            n691 = local write "Vg Array-Log-Used"(w1427) -> ()
            n692 = local write "Sat Id-Log-Used"(w1428) -> ()
            n693 = local write "Sat Id-Used"(w1434) -> ()
            n694 = local write "Index"(w1405) -> ()
            n695 = List Folder(path=w1398, error in=w1409) -> (filenames=w1441:string[], error out=w1408:errorcluster)  [unwired: 2 in, 2 out]
            n696 = Build Path(base path=w1398, name or relative path="ROI") -> (appended path=w1406:path)
            n697 = while {
              tunnel: w1441 -> [w1472]
              tunnel: w1405 -> [w1470]
              tunnel: [w1469] -> w1440
              tunnel: w1432 -> [w1468]
              i -> [w1469]
              stop <- w1465 stop-if-true
              n698 = Index Array(array=w1472, index=w1469) -> (element=w1473:string)
              n699 = xnode "Match Regular Expression"("input string"=w1473, "regular expression"=w1470) -> ("whole match"=w1471:string)  [unwired: 4 in, 4 out]
              n700 = Equal?(x=w1471, y=w1470) -> (x = y?=w1467:bool)
              n701 = Equal?(x=w1468, y=w1469) -> (x = y?=w1466:bool)
              n702 = Or(x=w1467, y=w1466) -> (x .or. y?=w1465:bool)
            }
            n703 = invoke on="Image Out" class="ImageControl" method="Clear ROI"(error in=w1408) -> (error out=w1412:errorcluster)  [unwired: 2 in, 2 out]
            n704 = Build Path(base path=w1406, name or relative path=w1405) -> (appended path=w1404:path)
            n705 = call <vilib>:"Check if File or Folder Exists.vi"("error in (no error)"=w1412, "path"=w1404) -> ("file or folder exists?"=w1410:bool, "dup path"=w1411:path)  [unwired: 7 in, 1 out]
            n706 = case shown="True" w1410 {
              tunnel: w1411 -> [_ w1460]
              frame False {
              }
              frame True {
                n707 = Read from Text File(file (use dialog)=w1460) -> (text=w1464:string)  [unwired: 3 in, 3 out]
                n708 = property on="Image Out" class="ImageControl"() -> ("ROI"=w1461:T10)  [unwired: 2 in, 2 out]
                n709 = Unflatten From String(type=w1461, binary string=w1464) -> (value=w1462:T10, error out=w1463:errorcluster)  [unwired: 3 in, 1 out]
                n710 = property on="Image Out" class="ImageControl"(error in=w1463, "ROI"=w1462) -> ()  [unwired: 1 in, 2 out]
              }
            }
            n711 = Index Array(array=w1441, index=w1440) -> (element=w1414:string)
            n712 = local write "Image Name"(w1414) -> ()
            n713 = Empty String/Path?(string/path=w1414) -> (empty?=w1421:bool)
            n714 = Build Path(base path=w1398, name or relative path=w1414) -> (appended path=w1413:path)
            n715 = local read "No Image"() -> (w1420:path)
            n716 = Select(t=w1420, s=w1421, f=w1413) -> (s? t:f=w1415:path)
            n717 = call <vilib>:"Get File Extension.vi"("file"=w1415) -> ("lowercase file extension"=w1417:string)  [unwired: 7 in, 3 out]
            n718 = local write "Image File"(w1415) -> ()
            n719 = local write "String"(w1417) -> ()
            n720 = Search 1D Array(1D array=string[] ["bmp", "jpeg", "png", "jpg", "gif"], element=w1417) -> (index of element=w1416:i32)  [unwired: 1 in]
            n721 = call "Vision Acquisition5"("Image Path"=w1415) -> ("Image Out"=w1419:T2)  [unwired: 25 in, 1 out]
            n722 = Less Than 0?(x=w1416) -> ()  [unwired: 1 out]
            n723 = local write "Image Out"(w1419) -> ()
            n724 = local write "Image Out 2"(w1419) -> ()
          }
          event "Save Changes? 3": Mouse Down {
            n725 = event-data() -> ()  [unwired: 1 in, 7 out]
            n726 = local read "Image Folder"() -> (w1589:path)
            n727 = Build Path(base path=w1589, name or relative path="ROI") -> (appended path=w1596:path)
            n728 = call <vilib>:"Check if File or Folder Exists.vi"("path"=w1596) -> ("file or folder exists?"=w1598:bool, "dup path"=w1595:path)  [unwired: 8 in, 1 out]
            n729 = case shown="False" w1598 {
              tunnel: w1595 -> [w1600 w1601]
              tunnel: [w1599 w1601] -> w1590
              frame False {
                n730 = Create Folder(path (use dialog)=w1600) -> (created path=w1599:path)  [unwired: 2 in, 2 out]
              }
              frame True {
              }
            }
            n731 = local read "Index"() -> (w1592:string)
            n732 = property on="Image Out" class="ImageControl"() -> ("ROI"=w1594:T10)  [unwired: 2 in, 2 out]
            n733 = Build Path(base path=w1590, name or relative path=w1592) -> (appended path=w1591:path)
            n734 = Flatten To String(anything=w1594) -> (data string=w1593:string)  [unwired: 3 in, 2 out]
            n735 = Write to Text File(file (use dialog)=w1591, text=w1593) -> ()  [unwired: 2 in, 3 out]
          }
          event "Next Button": Mouse Down {
            n736 = event-data() -> ()  [unwired: 1 in, 5 out]
            n737 = local read "XY Graph"() -> (w1614:cluster{dbl[], dbl[]}[])
            n738 = Decimate 1D Array(w1614) -> (w1610:cluster{dbl[], dbl[]}[], w1609:cluster{dbl[], dbl[]}[])
            n739 = Array To Cluster(array=w1610) -> (cluster=w1620:T9)
            n740 = local read "MobVi Index"() -> (w1616:dbl)
            n741 = Unbundle(w1620) -> ("[0]"=w1619:cluster{dbl[], dbl[]})  [unwired: 8 out]
            n742 = local read "NumPts"() -> (w1615:dbl)
            n743 = Unbundle(w1619) -> (w1618:dbl[], w1617:dbl[])
            n744 = local read "New: Dielectric"() -> (w1605:dbl)
            n745 = Increment(x=w1616) -> (x+1=w1611:dbl)
            n746 = local read "New: Length"() -> (w1604:dbl)
            n747 = local read "New: Width"() -> (w1603:dbl)
            n748 = local write "MobVi Index"(w1611) -> ()
            n749 = Array Subset(array=w1618, index=w1611, length=w1615) -> (w1607:dbl[])
            n750 = Array Subset(array=w1617, index=w1611, length=w1615) -> (w1606:dbl[])
            n751 = local write "Sat Vg Array-Used"(w1607) -> ()
            n752 = local write "Sat Id-Used"(w1606) -> ()
            n753 = call "Mobility-Vt-Used Pts_Saturation.vi"("Width"=w1603, "Length"=w1604, "Dielectric (d)"=w1605, "Sat Id Used"=w1606, "Vg Used"=w1607) -> ("Vt"=w1602:dbl, "Mobility"=w1608:dbl)  [unwired: 4 in, 1 out]
            n754 = Bundle(w1607, w1606) -> (w1613:cluster{dbl[], dbl[]})  [unwired: 1 in]
            n755 = Build Array (concatenate)(w1610, w1609, w1613) -> (w1612:cluster{dbl[], dbl[]}[])
            n756 = local write "New: Mobility-Sat"(w1608) -> ()
            n757 = local write "New: VT-Sat"(w1602) -> ()
            n758 = local write "XY Graph"(w1612) -> ()
          }
          event "Next Button 2": Mouse Down {
            n759 = event-data() -> ()  [unwired: 1 in, 7 out]
            n760 = local read "XY Graph 2"() -> (w1629:cluster{dbl[], dbl[]}[])
            n761 = Decimate 1D Array(w1629) -> (w1625:cluster{dbl[], dbl[]}[], w1624:cluster{dbl[], dbl[]}[])
            n762 = Array To Cluster(array=w1625) -> (cluster=w1635:T9)
            n763 = local read "Index 2"() -> (w1631:dbl)
            n764 = Unbundle(w1635) -> ("[0]"=w1634:cluster{dbl[], dbl[]})  [unwired: 8 out]
            n765 = local read "NumPts 2"() -> (w1630:dbl)
            n766 = Unbundle(w1634) -> (w1633:dbl[], w1632:dbl[])
            n767 = Increment(x=w1631) -> (x+1=w1626:dbl)
            n768 = local write "Index 2"(w1626) -> ()
            n769 = Array Subset(array=w1632, index=w1626, length=w1630) -> (w1621:dbl[])
            n770 = Array Subset(array=w1633, index=w1626, length=w1630) -> (w1622:dbl[])
            n771 = call "STS-Used.vi"("Id Used"=w1622, "Vg-Used"=w1621) -> ("STS"=w1623:dbl)  [unwired: 9 in]
            n772 = Bundle(w1622, w1621) -> (w1628:cluster{dbl[], dbl[]})  [unwired: 1 in]
            n773 = local write "Vg Array-Log-Used"(w1621) -> ()
            n774 = local write "Sat Id-Log-Used"(w1622) -> ()
            n775 = local write "New: STS"(w1623) -> ()
            n776 = Build Array (concatenate)(w1625, w1624, w1628) -> (w1627:cluster{dbl[], dbl[]}[])
            n777 = local write "XY Graph 2"(w1627) -> ()
          }
          event "Previous Button 2": Mouse Down {
            n778 = event-data() -> ()  [unwired: 1 in, 7 out]
            n779 = local read "XY Graph 2"() -> (w1645:cluster{dbl[], dbl[]}[])
            n780 = Decimate 1D Array(w1645) -> (w1642:cluster{dbl[], dbl[]}[], w1641:cluster{dbl[], dbl[]}[])
            n781 = Array To Cluster(array=w1642) -> (cluster=w1650:T9)
            n782 = local read "Index 2"() -> (w1638:dbl)
            n783 = Unbundle(w1650) -> ("[0]"=w1649:cluster{dbl[], dbl[]})  [unwired: 8 out]
            n784 = local read "NumPts 2"() -> (w1646:dbl)
            n785 = Unbundle(w1649) -> (w1648:dbl[], w1647:dbl[])
            n786 = Decrement(x=w1638) -> (x-1=w1639:dbl)
            n787 = local write "Index 2"(w1639) -> ()
            n788 = Array Subset(array=w1648, index=w1639, length=w1646) -> (w1636:dbl[])
            n789 = Array Subset(array=w1647, index=w1639, length=w1646) -> (w1637:dbl[])
            n790 = local write "Vg Array-Log-Used"(w1637) -> ()
            n791 = local write "Sat Id-Log-Used"(w1636) -> ()
            n792 = Bundle(w1636, w1637) -> (w1644:cluster{dbl[], dbl[]})  [unwired: 1 in]
            n793 = call "STS-Used.vi"("Id Used"=w1636, "Vg-Used"=w1637) -> ("STS"=w1640:dbl)  [unwired: 9 in]
            n794 = Build Array (concatenate)(w1642, w1641, w1644) -> (w1643:cluster{dbl[], dbl[]}[])
            n795 = local write "New: STS"(w1640) -> ()
            n796 = local write "XY Graph 2"(w1643) -> ()
          }
          event "Previous Button": Mouse Down {
            n797 = event-data() -> ()  [unwired: 1 in, 5 out]
            n798 = local read "XY Graph"() -> (w1664:cluster{dbl[], dbl[]}[])
            n799 = Decimate 1D Array(w1664) -> (w1661:cluster{dbl[], dbl[]}[], w1660:cluster{dbl[], dbl[]}[])
            n800 = Array To Cluster(array=w1661) -> (cluster=w1669:T9)
            n801 = local read "MobVi Index"() -> (w1659:dbl)
            n802 = Unbundle(w1669) -> ("[0]"=w1668:cluster{dbl[], dbl[]})  [unwired: 8 out]
            n803 = local read "NumPts"() -> (w1665:dbl)
            n804 = Unbundle(w1668) -> (w1667:dbl[], w1666:dbl[])
            n805 = Decrement(x=w1659) -> (x-1=w1658:dbl)
            n806 = local read "New: Dielectric"() -> (w1652:dbl)
            n807 = local read "New: Length"() -> (w1653:dbl)
            n808 = local read "New: Width"() -> (w1654:dbl)
            n809 = local write "MobVi Index"(w1658) -> ()
            n810 = Array Subset(array=w1667, index=w1658, length=w1665) -> (w1657:dbl[])
            n811 = Array Subset(array=w1666, index=w1658, length=w1665) -> (w1656:dbl[])
            n812 = local write "Sat Vg Array-Used"(w1657) -> ()
            n813 = local write "Sat Id-Used"(w1656) -> ()
            n814 = call "Mobility-Vt-Used Pts_Linear.vi"("Width"=w1654, "Length"=w1653, "Dielectric (d)"=w1652, "Sat Id Used"=w1656, "Vg Used"=w1657) -> ("Vt"=w1651:dbl, "Mobility"=w1655:dbl)  [unwired: 4 in, 1 out]
            n815 = Bundle(w1657, w1656) -> (w1663:cluster{dbl[], dbl[]})  [unwired: 1 in]
            n816 = local write "New: VT-Sat"(w1651) -> ()
            n817 = Build Array (concatenate)(w1661, w1660, w1663) -> (w1662:cluster{dbl[], dbl[]}[])
            n818 = local write "New: Mobility-Sat"(w1655) -> ()
            n819 = local write "XY Graph"(w1662) -> ()
          }
          event "Slide": Value Change {
            n820 = event-data() -> ()  [unwired: 1 in, 5 out]
            n821 = local read "XY Graph"() -> (w1682:cluster{dbl[], dbl[]}[])
            n822 = Decimate 1D Array(w1682) -> (w1679:cluster{dbl[], dbl[]}[], w1678:cluster{dbl[], dbl[]}[])
            n823 = Array To Cluster(array=w1679) -> (cluster=w1687:T9)
            n824 = Unbundle(w1687) -> ("[0]"=w1686:cluster{dbl[], dbl[]})  [unwired: 8 out]
            n825 = local read "NumPts"() -> (w1683:dbl)
            n826 = local read "Slide"() -> (w1671:dbl)
            n827 = Unbundle(w1686) -> (w1685:dbl[], w1684:dbl[])
            n828 = local read "New: Dielectric"() -> (w1672:dbl)
            n829 = local read "New: Length"() -> (w1673:dbl)
            n830 = local read "New: Width"() -> (w1674:dbl)
            n831 = local write "MobVi Index"(w1671) -> ()
            n832 = Array Subset(array=w1685, index=w1671, length=w1683) -> (w1677:dbl[])
            n833 = Array Subset(array=w1684, index=w1671, length=w1683) -> (w1676:dbl[])
            n834 = local write "Sat Vg Array-Used"(w1677) -> ()
            n835 = local write "Sat Id-Used"(w1676) -> ()
            n836 = call "Mobility-Vt-Used Pts_Linear.vi"("Width"=w1674, "Length"=w1673, "Dielectric (d)"=w1672, "Sat Id Used"=w1676, "Vg Used"=w1677) -> ("Vt"=w1670:dbl, "Mobility"=w1675:dbl)  [unwired: 4 in, 1 out]
            n837 = Bundle(w1677, w1676) -> (w1681:cluster{dbl[], dbl[]})  [unwired: 1 in]
            n838 = local write "New: VT-Sat"(w1670) -> ()
            n839 = Build Array (concatenate)(w1679, w1678, w1681) -> (w1680:cluster{dbl[], dbl[]}[])
            n840 = local write "New: Mobility-Sat"(w1675) -> ()
            n841 = local write "XY Graph"(w1680) -> ()
          }
          event "Slide 2": Value Change {
            n842 = event-data() -> ()  [unwired: 1 in, 5 out]
            n843 = local read "XY Graph 2"() -> (w1696:cluster{dbl[], dbl[]}[])
            n844 = Decimate 1D Array(w1696) -> (w1693:cluster{dbl[], dbl[]}[], w1692:cluster{dbl[], dbl[]}[])
            n845 = Array To Cluster(array=w1693) -> (cluster=w1701:T9)
            n846 = Unbundle(w1701) -> ("[0]"=w1700:cluster{dbl[], dbl[]})  [unwired: 8 out]
            n847 = local read "NumPts 2"() -> (w1697:dbl)
            n848 = local read "Slide 2"() -> (w1691:dbl)
            n849 = Unbundle(w1700) -> (w1699:dbl[], w1698:dbl[])
            n850 = local write "Index 2"(w1691) -> ()
            n851 = Array Subset(array=w1699, index=w1691, length=w1697) -> (w1689:dbl[])
            n852 = Array Subset(array=w1698, index=w1691, length=w1697) -> (w1688:dbl[])
            n853 = local write "Vg Array-Log-Used"(w1688) -> ()
            n854 = local write "Sat Id-Log-Used"(w1689) -> ()
            n855 = call "STS-Used.vi"("Id Used"=w1689, "Vg-Used"=w1688) -> ("STS"=w1690:dbl)  [unwired: 9 in]
            n856 = Bundle(w1689, w1688) -> (w1695:cluster{dbl[], dbl[]})  [unwired: 1 in]
            n857 = local write "New: STS"(w1690) -> ()
            n858 = Build Array (concatenate)(w1693, w1692, w1695) -> (w1694:cluster{dbl[], dbl[]}[])
            n859 = local write "XY Graph 2"(w1694) -> ()
          }
          event "Save Changes?": Mouse Down {
            n860 = event-data() -> ()  [unwired: 1 in, 5 out]
            n861 = flat-sequence {
              tunnel: [w1759] -> w1707
              tunnel: [w1758] -> w1705
              tunnel: [w1758] -> w1704
              tunnel: [w1708] -> w1702
              tunnel: w1707 -> [w1840]
              tunnel: [w1841] -> w1706
              tunnel: w1705 -> [w1841]
              tunnel: w1704 -> [w1839]
              tunnel: [w1837] -> w1703
              tunnel: w1702 -> [w1837]
              tunnel: w1706 -> [w1846]
              tunnel: w1703 -> [w1845]
              frame #0 {
                n862 = local read "Data File"() -> (w1759:path)
                n863 = call-poly <vilib>:"Read From Spreadsheet File.vi"("file path (dialog if empty)"=w1759) -> ("all rows"=w1711:string[][])  [unwired: 6 in, 4 out]
                n864 = flat-sequence {
                  tunnel: [w1794] -> w1756
                  tunnel: w1756 -> [w1811]
                  frame #0 {
                    # "Makes Empty File for Transformer Data"
                    n865 = local read "Data Folder"() -> (w1783:path)
                    n866 = Build Path(base path=w1783, name or relative path="Stats") -> (appended path=w1785:path)
                    n867 = call <vilib>:"Check if File or Folder Exists.vi"("path"=w1785) -> ("file or folder exists?"=w1786:bool, "dup path"=w1787:path)  [unwired: 8 in, 1 out]
                    n868 = case shown="False" w1786 {
                      tunnel: [w1791 w1793] -> w1788
                      tunnel: w1787 -> [w1792 w1793]
                      frame False {
                        n869 = Create Folder(path (use dialog)=w1792) -> (created path=w1791:path)  [unwired: 2 in, 2 out]
                      }
                      frame True {
                      }
                    }
                    n870 = Build Path(base path=w1788, name or relative path="Tranformer Data.txt") -> (appended path=w1790:path)
                    n871 = call-poly <vilib>:"Write To Spreadsheet File.vi"("append to file? (new file:F)"=TRUE, "file path (dialog if empty)"=w1790) -> ()  [unwired: 6 in, 1 out]
                  }
                  frame #1 {
                    # "Adds Headers if they don't exist"
                    n872 = Concatenate Strings("Stats\\", "Tranformer Data.txt") -> (w1801:string)
                    n873 = local read "Data Folder"() -> (w1800:path)
                    n874 = Build Path(base path=w1800, name or relative path=w1801) -> (appended path=w1794:path)
                    n875 = call-poly <vilib>:"Read From Spreadsheet File.vi"("file path (dialog if empty)"=w1794) -> ("first row"=w1799:string[])  [unwired: 6 in, 4 out]
                    n876 = Search 1D Array(1D array=w1799, element="DeviceID") -> (index of element=w1797:i32)  [unwired: 1 in]
                    n877 = Equal?(x=w1797, y=0) -> (x = y?=w1795:bool)
                    n878 = case shown="False" w1795 {
                      tunnel: w1794 -> [w1805 _]
                      frame False {
                        n879 = local read "Transformer \nHeaders"() -> (w1804:string[])
                        n880 = call-poly <vilib>:"Write To Spreadsheet File.vi"("1D data"=w1804, "file path (dialog if empty)"=w1805) -> ()  [unwired: 6 in, 1 out]
                      }
                      frame True {
                      }
                    }
                  }
                  frame #2 {
                    # "Adds current device if it doesn't exist"
                    n881 = local read "Current \nRecord"() -> (w1810:string[])
                    n882 = Index Array(array=w1810, index=0) -> (element=w1809:string)
                    n883 = Concatenate Strings("Stats\\", "Tranformer Data.txt") -> (w1814:string)
                    n884 = local read "Data Folder"() -> (w1813:path)
                    n885 = local write "Current Device ID"(w1809) -> ()
                    n886 = local read "Current Device ID"() -> (w1819:string)
                    n887 = Build Path(base path=w1813, name or relative path=w1814) -> (appended path=w1812:path)
                    n888 = call-poly <vilib>:"Read From Spreadsheet File.vi"("file path (dialog if empty)"=w1812) -> ("all rows"=w1806:string[][])  [unwired: 6 in, 4 out]
                    n889 = Index Array(array=w1806, index (col)=0) -> (element=w1807:string[])  [unwired: 1 in]
                    n890 = Search 1D Array(1D array=w1807, element=w1819) -> (index of element=w1808:i32)  [unwired: 1 in]
                    n891 = Equal?(x=w1808, y=-1) -> (x = y?=w1821:bool)
                    n892 = case shown="False" w1821 {
                      tunnel: w1811 -> [w1824 w1835]
                      tunnel: w1808 -> [w1827 _]
                      tunnel: w1806 -> [w1828 _]
                      frame False {
                        n893 = local read "Current \nRecord"() -> (w1826:string[])
                        n894 = Replace Array Subset(array=w1828, new element=w1826, index (row)=w1827) -> (w1825:string[][])  [unwired: 1 in]
                        n895 = flat-sequence {
                          tunnel: w1824 -> [w1829]
                          tunnel: w1825 -> [w1830]
                          tunnel: [w1830] -> w1823
                          tunnel: [w1829] -> w1822
                          tunnel: w1823 -> [w1832]
                          tunnel: w1822 -> [w1831]
                          frame #0 {
                            n896 = Delete(path (use dialog)=w1829) -> ()  [unwired: 4 in, 3 out]
                          }
                          frame #1 {
                            n897 = call-poly <vilib>:"Write To Spreadsheet File.vi"("append to file? (new file:F)"=TRUE, "2D data"=w1832, "file path (dialog if empty)"=w1831) -> ()  [unwired: 5 in, 1 out]
                          }
                        }
                      }
                      frame True {
                        n898 = local read "Current \nRecord"() -> (w1834:string[])
                        n899 = call-poly <vilib>:"Write To Spreadsheet File.vi"("append to file? (new file:F)"=TRUE, "1D data"=w1834, "file path (dialog if empty)"=w1835) -> ()  [unwired: 5 in, 1 out]
                      }
                    }
                  }
                }
                n900 = local read "New: Dielectric"() -> (w1749:dbl)
                n901 = local read "New: Mobility-Sat"() -> (w1741:dbl)
                n902 = Number To Fractional String(number=w1749) -> (F-format string=w1762:string)  [unwired: 3 in]
                n903 = local read "New: Temp"() -> (w1752:dbl)
                n904 = local read "New: STS"() -> (w1714:dbl)
                n905 = Number To Fractional String(number=w1741) -> (F-format string=w1737:string)  [unwired: 3 in]
                n906 = Number To Fractional String(number=w1714) -> (F-format string=w1717:string)  [unwired: 3 in]
                n907 = local read "New: Length"() -> (w1748:dbl)
                n908 = Replace Array Subset(array=w1711, new element=w1762, index (row)=7, index (col)=1) -> (w1766:string[][])
                n909 = local read "New: Width"() -> (w1750:dbl)
                n910 = local read "New: Length"() -> (w1771:dbl)
                n911 = Number To Decimal String(number=w1752) -> (decimal integer string=w1754:string)  [unwired: 1 in]
                n912 = local read "New: Trap Density-VT"() -> (w1722:dbl)
                n913 = local read "New: Mobility-Lin"() -> (w1730:dbl)
                n914 = Number To Fractional String(number=w1771) -> (F-format string=w1772:string)  [unwired: 3 in]
                n915 = Number To Fractional String(number=w1730) -> (F-format string=w1729:string)  [unwired: 3 in]
                n916 = Number To Fractional String(number=w1722) -> (F-format string=w1723:string)  [unwired: 3 in]
                n917 = local read "Index"() -> (w1774:string)
                n918 = Strip Path(path=w1759) -> (stripped path=w1779:path)  [unwired: 1 out]
                n919 = Number To Decimal String(number=w1748) -> (decimal integer string=w1769:string)  [unwired: 1 in]
                n920 = Number To Decimal String(number=w1750) -> (decimal integer string=w1770:string)  [unwired: 1 in]
                n921 = Concatenate Strings("_", w1754, "K") -> (w1751:string)
                n922 = Replace Array Subset(array=w1766, new element=w1772, index (row)=12, index (col)=1) -> (w1768:string[][])
                n923 = call "Build Text"("Temp"=w1751, "Index"=w1774, "Length"=w1769, "Width"=w1770) -> ("Result"=w1775:string)  [unwired: 10 in, 1 out]
                n924 = local read "New: Width"() -> (w1780:dbl)
                n925 = local read "New: VT-Sat"() -> (w1727:dbl)
                n926 = Number To Fractional String(number=w1780) -> (F-format string=w1760:string)  [unwired: 3 in]
                n927 = local read "New: Trap Density-VT"() -> (w1725:dbl)
                n928 = Number To Fractional String(number=w1727) -> (F-format string=w1739:string)  [unwired: 3 in]
                n929 = Number To Fractional String(number=w1725) -> (F-format string=w1716:string)  [unwired: 3 in]
                n930 = Path To String(path=w1779) -> (string=w1777:string)
                n931 = Replace Array Subset(array=w1768, new element=w1760, index (row)=13, index (col)=1) -> (w1767:string[][])
                n932 = Concatenate Strings(w1777, "\\", w1775) -> (w1776:string)
                n933 = local read "New: Temp"() -> (w1781:dbl)
                n934 = Number To Fractional String(number=w1781) -> (F-format string=w1761:string)  [unwired: 3 in]
                n935 = local read "New: VT-Lin"() -> (w1726:dbl)
                n936 = Number To Fractional String(number=w1726) -> (F-format string=w1738:string)  [unwired: 3 in]
                n937 = String To Path(string=w1776) -> (path=w1758:path)
                n938 = Replace Array Subset(array=w1767, new element=w1761, index (row)=14, index (col)=1) -> (w1710:string[][])
                n939 = Replace Array Subset(array=w1710, new element=w1737, index (row)=16, index (col)=1) -> (w1733:string[][])
                n940 = Replace Array Subset(array=w1733, new element=w1729, index (row)=17, index (col)=1) -> (w1731:string[][])
                n941 = Replace Array Subset(array=w1731, new element=w1739, index (row)=19, index (col)=1) -> (w1732:string[][])
                n942 = Replace Array Subset(array=w1732, new element=w1738, index (row)=20, index (col)=1) -> (w1709:string[][])
                n943 = Replace Array Subset(array=w1709, new element=w1717, index (row)=21, index (col)=1) -> (w1720:string[][])
                n944 = Replace Array Subset(array=w1720, new element=w1723, index (row)=22, index (col)=1) -> (w1721:string[][])
                n945 = Replace Array Subset(array=w1721, new element=w1716, index (row)=23, index (col)=1) -> (w1708:string[][])
              }
              frame #1 {
                n946 = Equal?(x=w1840, y=w1839) -> (x = y?=w1838:bool)
                n947 = case shown="False" w1838 {
                  tunnel: w1840 -> [w1844 _]
                  tunnel: w1839 -> [w1843 _]
                  frame False {
                    n948 = Move(source path=w1844, 9:TRUE, 10:w1843) -> ()  [unwired: 2 in, 3 out]
                  }
                  frame True {
                  }
                }
              }
              frame #2 {
                n949 = local write "Data File"(w1846) -> ()
                n950 = call-poly <vilib>:"Write To Spreadsheet File.vi"("2D data"=w1845, "file path (dialog if empty)"=w1846) -> ()  [unwired: 6 in, 1 out]
              }
            }
          }
          event "Save Changes? 2": Mouse Down {
            n951 = event-data() -> ()  [unwired: 1 in, 5 out]
            n952 = local read "Data File"() -> (w1870:path)
            n953 = call "Recorded Values.vi"("Path"=w1870) -> ("Recorded Char"=w1868:T5, "Recorded Prop"=w1867:T6, "Fabrication Prop"=w1869:T7)  [unwired: 8 in]
            n954 = Unbundle By Name(w1868) -> ("Mobility-Sat"=w1854:dbl, "Moblitity-Lin"=w1853:dbl, "On/Off"=w1852:dbl, "Threshold Voltage"=w1851:dbl, "STS"=w1850:dbl, "Trap Density-VT"=w1849:dbl, "Trap Density-STS"=w1848:dbl)  [unwired: 1 out]
            n955 = Unbundle By Name(w1867) -> ("Date Recorded"=w1859:string, "Index"=w1858:string, "Length"=w1857:dbl, "Width"=w1856:dbl, "Sample Temp"=w1855:dbl)
            n956 = Unbundle By Name(w1869) -> ("Date Created"=w1847:string, "Material"=w1866:string, "Solvent"=w1865:string, "Concentration"=w1864:dbl, "Method"=w1863:string, "Dielectric (nm)"=w1862:dbl, "Treatment"=w1861:string, "Comments"=w1860:string)
            n957 = local write "Rec: VT-Sat"(w1851) -> ()
            n958 = local write "Date Created"(w1847) -> ()
            n959 = local write "Rec: Material"(w1866) -> ()
            n960 = local write "Rec: Solvent"(w1865) -> ()
            n961 = local write "Rec: Concentration"(w1864) -> ()
            n962 = local write "Rec: Method"(w1863) -> ()
            n963 = local write "Rec: Dielectric (d)"(w1862) -> ()
            n964 = local write "Surface Treatment:"(w1861) -> ()
            n965 = local write "Comments"(w1860) -> ()
            n966 = local write "Index"(w1858) -> ()
            n967 = local write "Rec: Mobility-Sat"(w1854) -> ()
            n968 = local write "Rec: Mobility-Lin"(w1853) -> ()
            n969 = local write "Rec: On/Off"(w1852) -> ()
            n970 = local write "Rec: STS"(w1850) -> ()
            n971 = local write "Rec: Trap Density-VT"(w1849) -> ()
            n972 = local write "Rec: Trap Density-STS"(w1848) -> ()
            n973 = local write "Date Recorded"(w1859) -> ()
            n974 = local write "Rec: Length"(w1857) -> ()
            n975 = local write "Rec: Width"(w1856) -> ()
            n976 = local write "Rec: Temp"(w1855) -> ()
            n977 = stacked-sequence {
              seq-local: [w1928 _ _ _ _] -> [_ w2003 _ _ _]
              seq-local: [w1927 _ _ _ _] -> [_ w2004 _ _ _]
              seq-local: [w1928 _ _ _ _] -> [_ w2002 _ _ _]
              seq-local: [w1929 _ _ _ _] -> [_ w2000 _ _ _]
              seq-local: [_ w2004 _ _ _] -> [_ _ w2009 _ _]
              seq-local: [_ w2000 _ _ _] -> [_ _ w2008 _ _]
              frame #0 {
                n978 = local read "Data File"() -> (w1927:path)
                n979 = call-poly <vilib>:"Read From Spreadsheet File.vi"("file path (dialog if empty)"=w1927) -> ("all rows"=w1932:string[][])  [unwired: 6 in, 4 out]
                n980 = local read "New: Dielectric"() -> (w1970:dbl)
                n981 = local read "New: Mobility-Sat"() -> (w1962:dbl)
                n982 = Number To Fractional String(number=w1970) -> (F-format string=w1980:string)  [unwired: 3 in]
                n983 = local read "New: Temp"() -> (w1973:dbl)
                n984 = local read "New: STS"() -> (w1935:dbl)
                n985 = Number To Fractional String(number=w1962) -> (F-format string=w1958:string)  [unwired: 3 in]
                n986 = Number To Fractional String(number=w1935) -> (F-format string=w1938:string)  [unwired: 3 in]
                n987 = local read "New: Length"() -> (w1969:dbl)
                n988 = Replace Array Subset(array=w1932, new element=w1980, index (row)=7, index (col)=1) -> (w1984:string[][])
                n989 = local read "New: Width"() -> (w1971:dbl)
                n990 = local read "New: Length"() -> (w1989:dbl)
                n991 = Number To Decimal String(number=w1973) -> (decimal integer string=w1975:string)  [unwired: 1 in]
                n992 = local read "New: Trap Density-VT"() -> (w1943:dbl)
                n993 = local read "New: Mobility-Lin"() -> (w1951:dbl)
                n994 = Number To Fractional String(number=w1989) -> (F-format string=w1990:string)  [unwired: 3 in]
                n995 = Number To Fractional String(number=w1951) -> (F-format string=w1950:string)  [unwired: 3 in]
                n996 = Number To Fractional String(number=w1943) -> (F-format string=w1944:string)  [unwired: 3 in]
                n997 = local read "Index"() -> (w1992:string)
                n998 = Strip Path(path=w1927) -> (stripped path=w1997:path)  [unwired: 1 out]
                n999 = Number To Decimal String(number=w1969) -> (decimal integer string=w1987:string)  [unwired: 1 in]
                n1000 = Number To Decimal String(number=w1971) -> (decimal integer string=w1988:string)  [unwired: 1 in]
                n1001 = Concatenate Strings("_", w1975, "K") -> (w1972:string)
                n1002 = Replace Array Subset(array=w1984, new element=w1990, index (row)=12, index (col)=1) -> (w1986:string[][])
                n1003 = call "Build Text3"("Temp"=w1972, "Index"=w1992, "Length"=w1987, "Width"=w1988) -> ("Result"=w1993:string)  [unwired: 10 in, 1 out]
                n1004 = local read "New: Width"() -> (w1998:dbl)
                n1005 = local read "New: VT-Sat"() -> (w1948:dbl)
                n1006 = Number To Fractional String(number=w1998) -> (F-format string=w1978:string)  [unwired: 3 in]
                n1007 = local read "New: Trap Density-VT"() -> (w1946:dbl)
                n1008 = Number To Fractional String(number=w1948) -> (F-format string=w1960:string)  [unwired: 3 in]
                n1009 = Number To Fractional String(number=w1946) -> (F-format string=w1937:string)  [unwired: 3 in]
                n1010 = Path To String(path=w1997) -> (string=w1995:string)
                n1011 = Replace Array Subset(array=w1986, new element=w1978, index (row)=13, index (col)=1) -> (w1985:string[][])
                n1012 = Concatenate Strings(w1995, "\\", w1993) -> (w1994:string)
                n1013 = local read "New: Temp"() -> (w1999:dbl)
                n1014 = Number To Fractional String(number=w1999) -> (F-format string=w1979:string)  [unwired: 3 in]
                n1015 = local read "New: VT-Lin"() -> (w1947:dbl)
                n1016 = Number To Fractional String(number=w1947) -> (F-format string=w1959:string)  [unwired: 3 in]
                n1017 = String To Path(string=w1994) -> (path=w1928:path)
                n1018 = Replace Array Subset(array=w1985, new element=w1979, index (row)=14, index (col)=1) -> (w1931:string[][])
                n1019 = Replace Array Subset(array=w1931, new element=w1958, index (row)=16, index (col)=1) -> (w1954:string[][])
                n1020 = Replace Array Subset(array=w1954, new element=w1950, index (row)=17, index (col)=1) -> (w1952:string[][])
                n1021 = Replace Array Subset(array=w1952, new element=w1960, index (row)=19, index (col)=1) -> (w1953:string[][])
                n1022 = Replace Array Subset(array=w1953, new element=w1959, index (row)=20, index (col)=1) -> (w1930:string[][])
                n1023 = Replace Array Subset(array=w1930, new element=w1938, index (row)=21, index (col)=1) -> (w1941:string[][])
                n1024 = Replace Array Subset(array=w1941, new element=w1944, index (row)=22, index (col)=1) -> (w1942:string[][])
                n1025 = Replace Array Subset(array=w1942, new element=w1937, index (row)=23, index (col)=1) -> (w1929:string[][])
              }
              frame #1 {
                n1026 = Equal?(x=w2003, y=w2002) -> (x = y?=w2001:bool)
                n1027 = case shown="True" w2001 {
                  tunnel: w2003 -> [w2007 _]
                  tunnel: w2002 -> [w2006 _]
                  frame False {
                    n1028 = Move(source path=w2007, 9:TRUE, 10:w2006) -> ()  [unwired: 2 in, 3 out]
                  }
                  frame True {
                  }
                }
              }
              frame #2 {
                n1029 = local write "Data File"(w2009) -> ()
                n1030 = call-poly <vilib>:"Write To Spreadsheet File.vi"("2D data"=w2008, "file path (dialog if empty)"=w2009) -> ()  [unwired: 6 in, 1 out]
              }
              frame #3 {
                w2082 = 0
                # "Moves to next file and displays new image/data"
                n1031 = property on="Image Out" class="ImageControl"() -> (error out=w2044:errorcluster, "Image Center Position"=w2048:cluster{"X":u32, "Y":u32})  [unwired: 2 in, 1 out]
                n1032 = local read "Data File"() -> (w2087:path)
                n1033 = Strip Path(path=w2087) -> (stripped path=w2078:path, name=w2096:string)
                n1034 = Unbundle(w2048) -> ("X"=w2046:u32)  [unwired: 1 out]
                n1035 = local write "Data Folder"(w2078) -> ()
                n1036 = Bundle("X"=w2046, 0) -> (w2047:cluster{"X":u32, i32})  [unwired: 1 in]
                n1037 = property on="Image Out" class="ImageControl"(error in=w2044, "Image Center Position"=w2047) -> ()  [unwired: 1 in, 2 out]
                n1038 = List Folder(path=w2078) -> (filenames=w2092:string[])  [unwired: 3 in, 3 out]
                n1039 = Search 1D Array(1D array=w2092, element=w2096) -> (index of element=w2089:i32)  [unwired: 1 in]
                n1040 = Array Size(array=w2092) -> (size(s)=w2088:i32)
                n1041 = Decrement(x=w2088) -> (x-1=w2090:i32)
                n1042 = Equal?(x=w2089, y=w2090) -> (x = y?=w2091:bool)
                n1043 = local read "Folder Index"() -> (w2040:dbl)
                n1044 = case shown="False" w2091 {
                  tunnel: w2040 -> [w2219 _]
                  tunnel: [w2218 0] -> w2039
                  frame False {
                    n1045 = Increment(x=w2219) -> (x+1=w2218:dbl)
                  }
                  frame True {
                  }
                }
                n1046 = invoke on="Image Out" class="ImageControl" method="Clear ROI"() -> ()  [unwired: 3 in, 3 out]
                n1047 = local write "Folder Index"(w2039) -> ()
                n1048 = Path To String(path=w2078) -> (string=w2097:string)
                n1049 = Index Array(array=w2092, index=w2039) -> (element=w2093:string)
                n1050 = local write "Data Name:"(w2093) -> ()
                n1051 = Concatenate Strings(w2097, "\\", w2093) -> (w2095:string)
                n1052 = String To Path(string=w2095) -> (path=w2038:path)
                n1053 = local write "Data File"(w2038) -> ()
                n1054 = local read "NumPts 2"() -> (w2034:dbl)
                n1055 = local read "NumPts"() -> (w2023:dbl)
                n1056 = local read "NumPts"() -> (w2035:dbl)
                n1057 = call-poly <vilib>:"Read From Spreadsheet File.vi"("file path (dialog if empty)"=w2038) -> ("all rows"=w2084:string[][])  [unwired: 6 in, 4 out]
                n1058 = call "Mobility-Vt Calculator-File.vi"("NumPts"=w2035, "Path"=w2038) -> ("XY Graph-Sat"=w2036:cluster{dbl[], dbl[]}[], "XY Graph-Lin"=w2018:cluster{dbl[], dbl[]}[], "Output"=w2037:T8, "Index-Sat"=w2013:dbl, "Index-Lin"=w2022:dbl)  [unwired: 4 in, 1 out]
                n1059 = Decimate 1D Array(w2018) -> (w2030:cluster{dbl[], dbl[]}[])  [unwired: 1 out]
                n1060 = Array To Cluster(array=w2030) -> (cluster=w2028:T9)
                n1061 = Unbundle(w2028) -> ("[0]"=w2029:cluster{dbl[], dbl[]})  [unwired: 8 out]
                n1062 = local write "XY Graph-Lin"(w2018) -> ()
                n1063 = Unbundle(w2029) -> (w2027:dbl[], w2026:dbl[])
                n1064 = Array Subset(array=w2026, index=w2022, length=w2023) -> (w2024:dbl[])
                n1065 = Array Subset(array=w2027, index=w2022, length=w2023) -> (w2025:dbl[])
                n1066 = call "STS Calculator-File.vi"("NumPts"=w2034, "Path"=w2038) -> ("STS Index-Sat"=w2033:dbl, "XY Graph-Sat"=w2032:cluster{dbl[], dbl[]}[], "Ouput"=w2031:cluster{"STS-Sat":dbl, "STS-Lin":dbl})  [unwired: 5 in, 2 out]
                n1067 = local read "New: Dielectric"() -> (w2017:dbl)
                n1068 = local read "New: Temp"() -> (w2016:dbl)
                n1069 = local write "Lin Id-Used"(w2024) -> ()
                n1070 = local write "Lin-Vg Array-Used"(w2025) -> ()
                n1071 = local write "MobVi Index"(w2013) -> ()
                n1072 = local write "Slide"(w2013) -> ()
                n1073 = local write "XY Graph"(w2036) -> ()
                n1074 = local write "Index 2"(w2033) -> ()
                n1075 = local write "XY Graph 2"(w2032) -> ()
                n1076 = Unbundle By Name(w2037) -> ("Mobility-Sat"=w2021:dbl, "Vt-Sat"=w2012:dbl, "Mobility-Lin"=w2020:dbl, "Mobility-Lin"=w2019:dbl)
                n1077 = Array Size(array=w2084) -> (size(s)=w2083:i32[])
                n1078 = Unbundle By Name(w2031) -> ("STS-Sat"=w2015:dbl)
                n1079 = call "Trap Density_STS.vi"("Temp (T) [K]"=w2016, "S.T.S. (S)"=w2015, "Dielectric"=w2017) -> ("Trap Density (N)"=w2014:dbl)  [unwired: 8 in]
                n1080 = local write "Calc: Mobility-Sat"(w2021) -> ()
                n1081 = local write "Calc: Mobility-Lin"(w2019) -> ()
                n1082 = local write "New: Trap Density-STS"(w2014) -> ()
                n1083 = local read "Image Folder"() -> (w2072:path)
                n1084 = local write "Calc: VT-Sat"(w2012) -> ()
                n1085 = local write "Calc: VT-Lin"(w2020) -> ()
                n1086 = local read "New: Dielectric"() -> (w2010:dbl)
                n1087 = Decimate 1D Array(w2036) -> (w2067:cluster{dbl[], dbl[]}[])  [unwired: 1 out]
                n1088 = Index Array(array=w2083, index=w2082) -> (element=w2063:i32)
                n1089 = Decimate 1D Array(w2032) -> (w2057:cluster{dbl[], dbl[]}[])  [unwired: 1 out]
                n1090 = Array Subset(array=w2084, index (row)=w2082, index (col)=w2082, length (col)=3) -> (w2085:string[][])  [unwired: 1 in]
                n1091 = local write "Calc: STS"(w2015) -> ()
                n1092 = List Folder(path=w2072) -> (filenames=w2077:string[])  [unwired: 3 in, 3 out]
                n1093 = local write "New: Mobility-Sat"(w2021) -> ()
                n1094 = Array To Cluster(array=w2067) -> (cluster=w2069:T9)
                n1095 = Array To Cluster(array=w2057) -> (cluster=w2055:T9)
                n1096 = Reshape Array(w2085, w2063) -> (w2070:string[])
                n1097 = local write "New: Mobility-Lin"(w2020) -> ()
                n1098 = Subtract(x=w2063, y=20) -> (x-y=w2062:i32)
                n1099 = local write "New: VT-Sat"(w2012) -> ()
                n1100 = local write "New: VT-Lin"(w2019) -> ()
                n1101 = local write "New: STS"(w2015) -> ()
                n1102 = property on="Slide" class="Slide (strict)"("Scale.Maximum"=w2062) -> ()  [unwired: 2 in, 2 out]
                n1103 = call "Trap Density_VT.vi"("VT"=w2012, "Dielectric"=w2010) -> ("Trap Density-VT"=w2011:dbl)
                n1104 = Unbundle(w2069) -> ("[0]"=w2068:cluster{dbl[], dbl[]})  [unwired: 8 out]
                n1105 = Unbundle(w2055) -> ("[0]"=w2056:cluster{dbl[], dbl[]})  [unwired: 8 out]
                n1106 = Search 1D Array(1D array=w2070, element="Index:") -> (index of element=w2079:i32)  [unwired: 1 in]
                n1107 = local write "New: Trap Density-VT"(w2011) -> ()
                n1108 = Increment(x=w2079) -> (x+1=w2080:i32)
                n1109 = Unbundle(w2068) -> (w2059:dbl[], w2058:dbl[])
                n1110 = Unbundle(w2056) -> (w2054:dbl[], w2053:dbl[])
                n1111 = Array Subset(array=w2059, index=w2013, length=w2035) -> (w2066:dbl[])
                n1112 = Array Subset(array=w2058, index=w2013, length=w2035) -> (w2065:dbl[])
                n1113 = Array Subset(array=w2054, index=w2033, length=w2034) -> (w2061:dbl[])
                n1114 = Array Subset(array=w2053, index=w2033, length=w2034) -> (w2060:dbl[])
                n1115 = Index Array(array=w2070, index=w2080) -> (element=w2075:string)
                n1116 = local write "Vg Array-Log-Used"(w2060) -> ()
                n1117 = local write "Sat Id-Log-Used"(w2061) -> ()
                n1118 = local write "Sat Id-Used"(w2065) -> ()
                n1119 = local write "Index"(w2075) -> ()
                n1120 = local write "Sat Vg Array-Used"(w2066) -> ()
                n1121 = while {
                  tunnel: w2077 -> [w2105]
                  tunnel: w2075 -> [w2103]
                  tunnel: [w2102] -> _
                  tunnel: [w2102] -> w2076
                  tunnel: w2063 -> [w2101]
                  i -> [w2102]
                  stop <- w2098 stop-if-true
                  n1122 = Index Array(array=w2105, index=w2102) -> (element=w2106:string)
                  n1123 = xnode "Match Regular Expression"("input string"=w2106, "regular expression"=w2103) -> ("whole match"=w2104:string)  [unwired: 4 in, 4 out]
                  n1124 = Equal?(x=w2104, y=w2103) -> (x = y?=w2100:bool)
                  n1125 = Equal?(x=w2101, y=w2102) -> (x = y?=w2099:bool)
                  n1126 = Or(x=w2100, y=w2099) -> (x .or. y?=w2098:bool)
                }
                n1127 = Path To String(path=w2072) -> (string=w2074:string)
                n1128 = Index Array(array=w2077, index=w2076) -> (element=w2051:string)
                n1129 = local write "Image Name"(w2051) -> ()
                n1130 = Empty String/Path?(string/path=w2051) -> (empty?=w2052:bool)
                n1131 = Concatenate Strings(w2074, "\\", w2051) -> (w2073:string)
                n1132 = String To Path(string=w2073) -> (path=w2050:path)
                n1133 = local read "No Image"() -> (w2049:path)
                n1134 = Select(t=w2049, s=w2052, f=w2050) -> (s? t:f=w2043:path)
                n1135 = local write "Image File"(w2043) -> ()
                n1136 = local read "Image Out"() -> (w2041:T2)
                n1137 = call "IMAQ ReadFile"("File Path"=w2043, "Image"=w2041) -> ("Image Out"=w2042:T2)  [unwired: 5 in, 4 out]
                n1138 = local write "Image Out"(w2042) -> ()
                n1139 = local write "Image Out 2"(w2042) -> ()
              }
              frame #4 {
                # "Output ROI data"
                n1140 = local read "Image Folder"() -> (w2221:path)
                n1141 = Build Path(base path=w2221, name or relative path="ROI") -> (appended path=w2223:path)
                n1142 = local read "Index"() -> (w2222:string)
                n1143 = Build Path(base path=w2223, name or relative path=w2222) -> (appended path=w2228:path)
                n1144 = invoke on="Image Out" class="ImageControl" method="Clear ROI"() -> (error out=w2227:errorcluster)  [unwired: 3 in, 2 out]
                n1145 = call <vilib>:"Check if File or Folder Exists.vi"("error in (no error)"=w2227, "path"=w2228) -> ("file or folder exists?"=w2225:bool, "dup path"=w2226:path)  [unwired: 7 in, 1 out]
                n1146 = case shown="True" w2225 {
                  tunnel: w2226 -> [_ w2229]
                  frame False {
                  }
                  frame True {
                    n1147 = Read from Text File(file (use dialog)=w2229) -> (text=w2233:string)  [unwired: 3 in, 3 out]
                    n1148 = property on="Image Out" class="ImageControl"() -> ("ROI"=w2230:T10)  [unwired: 2 in, 2 out]
                    n1149 = Unflatten From String(type=w2230, binary string=w2233) -> (value=w2231:T10, error out=w2232:errorcluster)  [unwired: 3 in, 1 out]
                    n1150 = property on="Image Out" class="ImageControl"(error in=w2232, "ROI"=w2231) -> ()  [unwired: 1 in, 2 out]
                  }
                }
              }
            }
            n1151 = flat-sequence {
              tunnel: [w1884] -> w1871
              tunnel: w1871 -> [w1898]
              frame #0 {
                # "Makes Empty File for Transformer Data"
                n1152 = local read "Data Folder"() -> (w1873:path)
                n1153 = Build Path(base path=w1873, name or relative path="Stats") -> (appended path=w1875:path)
                n1154 = call <vilib>:"Check if File or Folder Exists.vi"("path"=w1875) -> ("file or folder exists?"=w1876:bool, "dup path"=w1877:path)  [unwired: 8 in, 1 out]
                n1155 = case shown="False" w1876 {
                  tunnel: [w1881 w1883] -> w1878
                  tunnel: w1877 -> [w1882 w1883]
                  frame False {
                    n1156 = Create Folder(path (use dialog)=w1882) -> (created path=w1881:path)  [unwired: 2 in, 2 out]
                  }
                  frame True {
                  }
                }
                n1157 = Build Path(base path=w1878, name or relative path="Tranformer Data.txt") -> (appended path=w1880:path)
                n1158 = call-poly <vilib>:"Write To Spreadsheet File.vi"("append to file? (new file:F)"=TRUE, "file path (dialog if empty)"=w1880) -> ()  [unwired: 6 in, 1 out]
              }
              frame #1 {
                # "Adds Headers if they don't exist"
                n1159 = Concatenate Strings("Stats\\", "Tranformer Data.txt") -> (w1891:string)
                n1160 = local read "Data Folder"() -> (w1890:path)
                n1161 = Build Path(base path=w1890, name or relative path=w1891) -> (appended path=w1884:path)
                n1162 = call-poly <vilib>:"Read From Spreadsheet File.vi"("file path (dialog if empty)"=w1884) -> ("first row"=w1889:string[])  [unwired: 6 in, 4 out]
                n1163 = Search 1D Array(1D array=w1889, element="DeviceID") -> (index of element=w1887:i32)  [unwired: 1 in]
                n1164 = Equal?(x=w1887, y=0) -> (x = y?=w1885:bool)
                n1165 = case shown="False" w1885 {
                  tunnel: w1884 -> [w1895 _]
                  frame False {
                    n1166 = local read "Transformer \nHeaders"() -> (w1894:string[])
                    n1167 = call-poly <vilib>:"Write To Spreadsheet File.vi"("1D data"=w1894, "file path (dialog if empty)"=w1895) -> ()  [unwired: 6 in, 1 out]
                  }
                  frame True {
                  }
                }
              }
              frame #2 {
                # "Adds current device if it doesn't exist"
                n1168 = local read "Current \nRecord"() -> (w1901:string[])
                n1169 = Index Array(array=w1901, index=0) -> (element=w1900:string)
                n1170 = Concatenate Strings("Stats\\", "Tranformer Data.txt") -> (w1904:string)
                n1171 = local read "Data Folder"() -> (w1903:path)
                n1172 = local write "Current Device ID"(w1900) -> ()
                n1173 = local read "Current Device ID"() -> (w1910:string)
                n1174 = Build Path(base path=w1903, name or relative path=w1904) -> (appended path=w1902:path)
                n1175 = call-poly <vilib>:"Read From Spreadsheet File.vi"("file path (dialog if empty)"=w1902) -> ("all rows"=w1897:string[][])  [unwired: 6 in, 4 out]
                n1176 = Index Array(array=w1897, index (col)=0) -> (element=w1908:string[])  [unwired: 1 in]
                n1177 = Search 1D Array(1D array=w1908, element=w1910) -> (index of element=w1896:i32)  [unwired: 1 in]
                n1178 = Equal?(x=w1896, y=-1) -> (x = y?=w1899:bool)
                n1179 = case shown="False" w1899 {
                  tunnel: w1898 -> [w1912 w1925]
                  tunnel: w1896 -> [w1917 _]
                  tunnel: w1897 -> [w1918 _]
                  frame False {
                    n1180 = local read "Current \nRecord"() -> (w1916:string[])
                    n1181 = Replace Array Subset(array=w1918, new element=w1916, index (row)=w1917) -> (w1913:string[][])  [unwired: 1 in]
                    n1182 = flat-sequence {
                      tunnel: [w1919] -> _
                      tunnel: [w1920] -> _
                      tunnel: [w1920] -> w1915
                      tunnel: [w1919] -> w1914
                      tunnel: w1913 -> [w1920]
                      tunnel: w1912 -> [w1919]
                      tunnel: w1915 -> [w1922]
                      tunnel: w1914 -> [w1921]
                      frame #0 {
                        n1183 = Delete(path (use dialog)=w1919) -> ()  [unwired: 4 in, 3 out]
                      }
                      frame #1 {
                        n1184 = call-poly <vilib>:"Write To Spreadsheet File.vi"("append to file? (new file:F)"=TRUE, "2D data"=w1922, "file path (dialog if empty)"=w1921) -> ()  [unwired: 5 in, 1 out]
                      }
                    }
                  }
                  frame True {
                    n1185 = local read "Current \nRecord"() -> (w1924:string[])
                    n1186 = call-poly <vilib>:"Write To Spreadsheet File.vi"("append to file? (new file:F)"=TRUE, "1D data"=w1924, "file path (dialog if empty)"=w1925) -> ()  [unwired: 5 in, 1 out]
                  }
                }
              }
            }
          }
          event "Export": Mouse Down {
            n1187 = event-data() -> ()  [unwired: 1 in, 7 out]
            n1188 = call "OA_ConnectToOrigin.vi"() -> ("error out"=w2255:errorcluster, "Origin.IOApplication"=w2256:refnum<k7>)  [unwired: 8 in]
            n1189 = local read "Data Folder"() -> (w2234:path)
            n1190 = local read "Project"() -> (w2254:path)
            n1191 = call "OA_Load.vi"("error in (no error)"=w2255, "Path"=w2254, "Origin.IOApplication"=w2256) -> ("error out"=w2247:errorcluster, "Origin.IOApplication"=w2248:refnum<k7>)  [unwired: 1 out]
            n1192 = call "OAExecute.vi"("script"="document -m 3;", "Error IO"=w2247, "Origin.IOApplication"=w2248) -> ("Error IO Out"=w2245:errorcluster, "Origin.IOApplication"=w2246:refnum<k7>)  [unwired: 1 in, 1 out]
            n1193 = Build Path(base path=w2234, name or relative path="Stats") -> (appended path=w2235:path)
            n1194 = flat-sequence {
              tunnel: w2234 -> [w2276]
              tunnel: w2253 -> [w2275]
              tunnel: [w2265] -> w2258
              tunnel: [w2266] -> w2257
              tunnel: w2246 -> [w2270]
              tunnel: w2245 -> [w2269]
              tunnel: w2234 -> [w2292]
              tunnel: w2253 -> [w2291]
              tunnel: w2258 -> [w2287]
              tunnel: w2257 -> [w2288]
              tunnel: [w2282] -> w2252
              tunnel: [w2281] -> w2251
              tunnel: w2234 -> [w2303]
              tunnel: w2253 -> [w2302]
              tunnel: w2252 -> [w2298]
              tunnel: w2251 -> [w2297]
              tunnel: [w2296] -> w2250
              tunnel: [w2295] -> w2249
              tunnel: w2234 -> [w2318]
              tunnel: w2253 -> [w2317]
              tunnel: w2250 -> [w2312]
              tunnel: w2249 -> [w2311]
              tunnel: [w2309] -> w2243
              tunnel: [w2308] -> w2242
              frame #0 {
                n1195 = call "Param_Analysis.vi"("error in (no error)"=w2269, "Folder 2"=w2276, "Parameter String"="Mobility (cm^2/Vs):", "Parameter Name"="Mobility", "Folder"=w2275) -> ("error out"=w2272:errorcluster, "Array 4"=w2262:string[], "Array 3"=w2271:string[][])  [unwired: 3 in, 1 out]
                n1196 = call "Origin_Export.vi"("String 3"="[MobHistTab]Sheet1", "error in (no error)"=w2272, "Array"=w2271, "String 2"="[MOBvsLTable]Mobilities", "String"="pe_cd \"Mobility Chart\";", "Origin.IOApplication"=w2270, "Array 2"=w2262) -> ("reference out"=w2268:refnum<k7>, "error out"=w2267:errorcluster)  [unwired: 2 in, 1 out]
                n1197 = call "OAExecute.vi"("script"="window -a MOBvsLTable;\nwindow -s TV;", "Error IO"=w2267, "Origin.IOApplication"=w2268) -> ("Error IO Out"=w2265:errorcluster, "Origin.IOApplication"=w2266:refnum<k7>)  [unwired: 1 in, 1 out]
              }
              frame #1 {
                n1198 = call "Param_Analysis.vi"("error in (no error)"=w2287, "Folder 2"=w2292, "Parameter String"="On/Off Current:", "Parameter Name"="On_Off_Current", "Folder"=w2291) -> ("error out"=w2286:errorcluster, "Array 4"=w2280:string[], "Array 3"=w2283:string[][])  [unwired: 3 in, 1 out]
                n1199 = call "Origin_Export.vi"("String 3"="[OnOffHistTab]Sheet1", "error in (no error)"=w2286, "Array"=w2283, "String 2"="[OnOffTable]On/Off Ratios", "String"="pe_cd \"OnOff vs L\";", "Origin.IOApplication"=w2288, "Array 2"=w2280) -> ("reference out"=w2282:refnum<k7>, "error out"=w2281:errorcluster)  [unwired: 2 in, 1 out]
              }
              frame #2 {
                n1200 = call "Param_Analysis.vi"("Folder 2"=w2303, "Parameter String"="S.T.S. (V/decade):", "Parameter Name"="STS", "Folder"=w2302) -> ("Array 4"=w2294:string[], "Array 3"=w2299:string[][])  [unwired: 4 in, 2 out]
                n1201 = call "Origin_Export.vi"("String 3"="[SHistTab]Sheet1", "error in (no error)"=w2297, "Array"=w2299, "String 2"="[STable]Threshold Swing", "String"="pe_cd \"Threshold Swing vs L\";", "Origin.IOApplication"=w2298, "Array 2"=w2294) -> ("reference out"=w2295:refnum<k7>, "error out"=w2296:errorcluster)  [unwired: 2 in, 1 out]
              }
              frame #3 {
                n1202 = call "Param_Analysis.vi"("Folder 2"=w2318, "Parameter String"="Threshold V (V):", "Parameter Name"="Threshold_V", "Folder"=w2317) -> ("Array 4"=w2307:string[], "Array 3"=w2310:string[][])  [unwired: 4 in, 2 out]
                n1203 = call "Origin_Export.vi"("String 3"="[VtHistTab]Sheet1", "error in (no error)"=w2312, "Array"=w2310, "String 2"="[VtTable]Threshold Voltages", "String"="pe_cd \"Threshold Voltage vs L\";", "Origin.IOApplication"=w2311, "Array 2"=w2307) -> ("reference out"=w2309:refnum<k7>, "error out"=w2308:errorcluster)  [unwired: 2 in, 1 out]
              }
            }
            n1204 = call <vilib>:"Check if File or Folder Exists.vi"("path"=w2235) -> ("file or folder exists?"=w2260:bool, "dup path"=w2259:path)  [unwired: 8 in, 1 out]
            n1205 = case shown="False" w2260 {
              tunnel: w2259 -> [w2320 w2321]
              tunnel: [w2319 w2321] -> w2253
              frame False {
                n1206 = Create Folder(path (use dialog)=w2320) -> (created path=w2319:path)  [unwired: 2 in, 2 out]
              }
              frame True {
              }
            }
            n1207 = call "File Dialog"("start path"=w2235) -> ("selected path"=w2238:path)  [unwired: 11 in, 3 out]
            n1208 = Path To String(path=w2238) -> (string=w2237:string)
            n1209 = call "OAExecute.vi"("script"="pe_cd /;\npe_cd \"Mobility Chart\"; ", "Error IO"=w2242, "Origin.IOApplication"=w2243) -> ("Error IO Out"=w2239:errorcluster, "Origin.IOApplication"=w2240:refnum<k7>)  [unwired: 1 in, 1 out]
            n1210 = call "OASaveProject.vi"("path"=w2237, "Error IO"=w2239, "Origin.IOApplication"=w2240) -> ()  [unwired: 3 out]
          }
          event "Blank Button": Mouse Down {
            n1211 = event-data() -> ()  [unwired: 1 in, 7 out]
            n1212 = local read "Data File"() -> (w2329:path)
            n1213 = Strip Path(path=w2329) -> (stripped path=w2325:path, name=w2327:string)
            n1214 = Path To String(path=w2325) -> (string=w2324:string)
            n1215 = Concatenate Strings(w2324, "\\", "X_", w2327) -> (w2323:string)
            n1216 = String To Path(string=w2323) -> (path=w2322:path)
            n1217 = Move(source path=w2329, 10:w2322) -> ()  [unwired: 3 in, 3 out]
            n1218 = local write "Data File"(w2322) -> ()
          }
          event "Cancel Button": Mouse Down {
            (unwired) 6
            n1219 = event-data() -> ()  [unwired: 1 in, 7 out]
            n1220 = call "Simulate_Keyboard.vi"("Action"=2, "Virtual Key"=162) -> ()  [unwired: 7 in, 1 out]
          }
        }
        n1221 = Reciprocal(x=w515) -> (1/x=w514:sgl)
        n1222 = Multiply(x=w514, y=10) -> (x*y=w516:sgl)
        n1223 = case shown="\"EQUALS\"" w555 {
          tunnel: w529 -> [w606 w612 w616 w618 w622 w624 w626 w628 w630 w632 w634 w636 w638 w640 w642 w644 w646 w648 w650 w652 w654 w656 w658 w660 w662 w664 w666 w668 w670 w672 w674 w676 w678 w680 w682 w684 w686 w688 w690 w692 w694 w696 w698 w700 w702 w704 w706 w708 w710 w712 w714 w716 w718 w720 w722 w724 w726 w728 w730 w732 w734 w736 w738 w740 w742 w744 w746 w748 w750 w752 w754 w756 w758 w760 w762 w764 w766 w768 w770 w772 w774 w776 w778 w780 w782 w784 w786 w788 w790 w792 w794 w796 w798 w800 w802 w804 w806 w808 w810 w812 w814 w816 w818 w820 w822]
          tunnel: [w606 w611 w615 w618 w622 w624 w626 w628 w630 w632 w634 w636 w638 w640 w642 w644 w646 w648 w650 w652 w654 w656 w658 w660 w662 w664 w666 w668 w670 w672 w674 w676 w678 w680 w682 w684 w686 w688 w690 w692 w694 w696 w698 w700 w702 w704 w706 w708 w710 w712 w714 w716 w718 w720 w722 w724 w726 w728 w730 w732 w734 w736 w738 w740 w742 w744 w746 w748 w750 w752 w754 w756 w758 w760 w762 w764 w766 w768 w770 w772 w774 w776 w778 w780 w782 w784 w786 w788 w790 w792 w794 w796 w798 w800 w802 w804 w806 w808 w810 w812 w814 w816 w818 w820 w822] -> w554
          tunnel: w530 -> [w608 w610 w614 w620 w621 w623 w625 w627 w629 w631 w633 w635 w637 w639 w641 w643 w645 w647 w649 w651 w653 w655 w657 w659 w661 w663 w665 w667 w669 w671 w673 w675 w677 w679 w681 w683 w685 w687 w689 w691 w693 w695 w697 w699 w701 w703 w705 w707 w709 w711 w713 w715 w717 w719 w721 w723 w725 w727 w729 w731 w733 w735 w737 w739 w741 w743 w745 w747 w749 w751 w753 w755 w757 w759 w761 w763 w765 w767 w769 w771 w773 w775 w777 w779 w781 w783 w785 w787 w789 w791 w793 w795 w797 w799 w801 w803 w805 w807 w809 w811 w813 w815 w817 w819 w821]
          tunnel: [w607 w610 w614 w619 w621 w623 w625 w627 w629 w631 w633 w635 w637 w639 w641 w643 w645 w647 w649 w651 w653 w655 w657 w659 w661 w663 w665 w667 w669 w671 w673 w675 w677 w679 w681 w683 w685 w687 w689 w691 w693 w695 w697 w699 w701 w703 w705 w707 w709 w711 w713 w715 w717 w719 w721 w723 w725 w727 w729 w731 w733 w735 w737 w739 w741 w743 w745 w747 w749 w751 w753 w755 w757 w759 w761 w763 w765 w767 w769 w771 w773 w775 w777 w779 w781 w783 w785 w787 w789 w791 w793 w795 w797 w799 w801 w803 w805 w807 w809 w811 w813 w815 w817 w819 w821] -> w553
          tunnel: w516 -> [w605 w609 w613 w617 _ _ _ _ _ _ _ _ _ _ _ _ _ _ _ _ _ _ _ _ _ _ _ _ _ _ _ _ _ _ _ _ _ _ _ _ _ _ _ _ _ _ _ _ _ _ _ _ _ _ _ _ _ _ _ _ _ _ _ _ _ _ _ _ _ _ _ _ _ _ _ _ _ _ _ _ _ _ _ _ _ _ _ _ _ _ _ _ _ _ _ _ _ _ _ _ _ _ _ _ _]
          frame "DOWN" {
            n1224 = Add(x=w608, y=w605) -> (x+y=w607:sgl)
          }
          frame "LEFT" {
            n1225 = Subtract(x=w612, y=w609) -> (x-y=w611:sgl)
          }
          frame "RIGHT" {
            n1226 = Add(x=w616, y=w613) -> (x+y=w615:sgl)
          }
          frame "UP" {
            n1227 = Subtract(x=w620, y=w617) -> (x-y=w619:sgl)
          }
          frame "ENTER (num pad)" {
          }
          frame "' (quote)" {
          }
          frame "END" {
          }
          frame "EQUALS" {
          }
          frame "ESCAPE" {
          }
          frame "GRAVE (`)" {
          }
          frame "HOME" {
          }
          frame "INSERT" {
          }
          frame "LBRACKET" {
          }
          frame "LCONTROL" {
          }
          frame "L ALT" {
          }
          frame "LSHIFT" {
          }
          frame "LWIN" {
          }
          frame "MINUS" {
          }
          frame "MULTIPLY" {
          }
          frame "NEXT" {
          }
          frame "NUMLOCK" {
          }
          frame "NUMPAD_0" {
          }
          frame "NUMPAD_1" {
          }
          frame "NUMPAD_2" {
          }
          frame "NUMPAD_3" {
          }
          frame "NUMPAD_4" {
          }
          frame "NUMPAD_5" {
          }
          frame "NUMPAD_6" {
          }
          frame "NUMPAD_7" {
          }
          frame "NUMPAD_8" {
          }
          frame "NUMPAD_9" {
          }
          frame "PAUSE" {
          }
          frame "PERIOD" {
          }
          frame "PRIOR (PG UP)" {
          }
          frame "RBRACKET" {
          }
          frame "RCONTROL" {
          }
          frame "RETURN" {
          }
          frame "R ALT" {
          }
          frame "RSHIFT" {
          }
          frame "RWIN" {
          }
          frame "SCROLL" {
          }
          frame "SEMICOLON" {
          }
          frame "SLASH" {
          }
          frame "SPACE" {
          }
          frame "SUBTRACT" {
          }
          frame "TAB" {
          }
          frame "DIVIDE" {
          }
          frame "DELETE" {
          }
          frame "DECIMAL" {
          }
          frame "COMMA" {
          }
          frame "CAPITAL" {
          }
          frame "BACKSLASH" {
          }
          frame "BACK" {
          }
          frame "ADD" {
          }
          frame "F15" {
          }
          frame "F14" {
          }
          frame "F13" {
          }
          frame "F12" {
          }
          frame "F11" {
          }
          frame "F10" {
          }
          frame "F9" {
          }
          frame "F8" {
          }
          frame "F7" {
          }
          frame "F6" {
          }
          frame "F5" {
          }
          frame "F4" {
          }
          frame "F3" {
          }
          frame "F2" {
          }
          frame "F1" {
          }
          frame "Z" {
          }
          frame "Y" {
          }
          frame "X" {
          }
          frame "W" {
          }
          frame "V" {
          }
          frame "U" {
          }
          frame "T" {
          }
          frame "S" {
          }
          frame "R" {
          }
          frame "Q" {
          }
          frame "P" {
          }
          frame "O" {
          }
          frame "N" {
          }
          frame "M" {
          }
          frame "L" {
          }
          frame "K" {
          }
          frame "J" {
          }
          frame "I" {
          }
          frame "H" {
          }
          frame "G" {
          }
          frame "F" {
          }
          frame "E" {
          }
          frame "D" {
          }
          frame "C" {
          }
          frame "B" {
          }
          frame "A" {
          }
          frame "9" {
          }
          frame "8" {
          }
          frame "7" {
          }
          frame "6" {
          }
          frame "5" {
          }
          frame "4" {
          }
          frame "3" {
          }
          frame "2" {
          }
          frame "1" {
          }
          frame "0" {
          }
        }
        n1228 = Bundle(w532, w531, w546, w545, 0.0) -> (w544:cluster{dbl, dbl, dbl, dbl, dbl})  [unwired: 1 in]
        n1229 = Bundle("X"=w554, "Y"=w553) -> (w548:cluster{"X":sgl, "Y":sgl})  [unwired: 1 in]
        n1230 = Divide(x=20, y=w515) -> (x/y=w518:sgl)
        n1231 = property on="Image Out" class="ImageControl"("Image Center Position"=w548) -> ()  [unwired: 2 in, 2 out]
        n1232 = call "IMAQ Convert Rectangle to ROI (Polygon)"("Rectangle"=w544) -> ("ROI Descriptor"=w542:T3)  [unwired: 7 in, 2 out]
        n1233 = Bundle("Application Font", w518, w522, w522, w522, w522, w522, TRUE, w520) -> (w524:T16)  [unwired: 1 in]
        n1234 = property on="Image Out 2" class="ImageControl"("ROI"=w542) -> ()  [unwired: 2 in, 2 out]
        n1235 = Bundle(w520, w524, w520, w520) -> (w523:T17)  [unwired: 1 in]
        n1236 = property on="Image Out" class="ImageControl"() -> ("ROI"=w507:T10)  [unwired: 2 in, 2 out]
        n1237 = Unbundle By Name(w507) -> ("Contours"=w571:T14)
        n1238 = local read "Image Out"() -> (w526:T2)
        n1239 = call "IMAQ Clear Overlay"("Image"=w526) -> ("Image Out"=w525:T2)  [unwired: 9 in, 1 out]
        n1240 = Initialize Array(0) -> (w569:i32[])  [unwired: 1 in]
        n1241 = local read "Magnification"() -> (w560:u16)
        n1242 = Array Size(array=w571) -> (size(s)=w570:i32)
        n1243 = Build Array(0.505025, 0.252522, 0.127742, 0.050345, 0.031129) -> (w561:dbl[])
        n1244 = Array Subset(array=w561, index=w560, length=1) -> (w558:dbl[])
        n1245 = property on="Image Out" class="ImageControl"() -> ("ZoomInteger"=w550:cluster{"X":i32, "Y":i32})  [unwired: 2 in, 2 out]
        n1246 = To Double Precision Float(number=w558) -> (double precision float=w557:dbl[])
        n1247 = for {
          N: w570 -> [_]
          shift-right: [w845] -> _
          shift-left: w571 -> [w845]
          shift-right: [w843] -> w556
          shift-left: w569 -> [w842]
          tunnel: w557 -> [w841]
          shift-right: [w838] -> _
          shift-left: w525 -> [w840]
          tunnel: w523 -> [w833]
          i -> [w837]
          n1248 = Index Array(array=w845, index=w837) -> (element=w854:T18)
          n1249 = Unbundle(w854) -> ("Points"=w853:i32[])  [unwired: 2 out]
          n1250 = Array To Cluster(array=w853) -> (cluster=w852:T19)
          n1251 = Unbundle(w852) -> ("Points[0]"=w832:i32, "Points[1]"=w829:i32, "Points[2]"=w844:i32, "Points[3]"=w850:i32)  [unwired: 5 out]
          n1252 = Add(x=w832, y=10) -> (x+y=w830:i32)
          n1253 = Subtract(x=w829, y=w850) -> (x-y=w849:i32)
          n1254 = Subtract(x=w832, y=w844) -> (x-y=w851:i32)
          n1255 = Square(x=w849) -> (x^2=w847:i32)
          n1256 = Square(x=w851) -> (x^2=w848:i32)
          n1257 = Add(x=w848, y=w847) -> (x+y=w846:i32)
          n1258 = Square Root(x=w846) -> (sqrt(x)=w823:dbl)
          n1259 = Multiply(x=w823, y=0.5) -> (x*y=w826:dbl)
          n1260 = Add(x=w826, y=w829) -> (x+y=w828:dbl)
          n1261 = Bundle(w830, w828) -> (w839:cluster{i32, dbl})  [unwired: 1 in]
          n1262 = Multiply(x=w823, y=w841) -> (x*y=w836:dbl[])
          n1263 = Index Array(array=w836) -> (element=w835:dbl)  [unwired: 1 in]
          n1264 = Number To Fractional String(number=w835) -> (F-format string=w834:string)  [unwired: 3 in]
          n1265 = call "IMAQ Overlay Text"("BG Color (Transparent)"=u32 0, "Text Color (black)"=u32 16448250, "Font, Size & Style"=w833, "String"=w834, "Origin"=w839, "Image"=w840) -> ("Image Out"=w838:T2)  [unwired: 4 in, 1 out]
          n1266 = Build Array (concatenate)(w842, w836) -> (w843:dbl[])
          n1267 = local write "Numeric 3"(w823) -> ()
        }
        n1268 = local write "ROI Descriptor"(w507) -> ()
        n1269 = Unbundle(w550) -> ("X"=w549:i32)  [unwired: 1 out]
        n1270 = Add Array Elements(numeric array=w556) -> (sum=w567:dbl)
        n1271 = local write "Distances"(w556) -> ()
        n1272 = local write "Total Width"(w567) -> ()
        n1273 = local write "Zoom"(w549) -> ()
        n1274 = local read "Total Width"() -> (w510:dbl)
        n1275 = local read "Rec: Width"() -> (w508:dbl)
        n1276 = local read "Manual-Width"() -> (w506:bool)
        n1277 = Not(x=w506) -> (.not. x?=w504:bool)
        n1278 = Equal To 0?(x=w510) -> (x = 0?=w505:bool)
        n1279 = Or(x=w505, y=w506) -> (x .or. y?=w509:bool)
        n1280 = And(x=w505, y=w504) -> (x .and. y?=w503:bool)
        n1281 = case shown="True" w503 {
          tunnel: w508 -> [_ w583]
          frame False {
          }
          frame True {
            n1282 = local write "New: Width"(w583) -> ()
          }
        }
        n1283 = case shown="False" w509 {
          tunnel: w510 -> [w584 _]
          frame False {
            n1284 = local write "New: Width"(w584) -> ()
          }
          frame True {
          }
        }
        n1285 = local read "Manuel-Dielectric"() -> (w432:bool)
        n1286 = local read "Rec: Dielectric (d)"() -> (w431:dbl)
        n1287 = local read "Manuel-Length"() -> (w433:bool)
        n1288 = local read "Rec: Length"() -> (w434:dbl)
        n1289 = case shown="False" w433 {
          tunnel: w434 -> [w574 _]
          frame False {
            n1290 = local write "New: Length"(w574) -> ()
          }
          frame True {
          }
        }
        n1291 = case shown="False" w432 {
          tunnel: w431 -> [w573 _]
          frame False {
            n1292 = local write "New: Dielectric"(w573) -> ()
          }
          frame True {
          }
        }
      }
    }
  }
  n1293 = Build Array("DeviceID", "Fabricator", "Deposition", "Date", "Sample", "Row", "Column", "L (um)", "W (um)", "Material", "Treatment", "TC (mM)", "Solvent", "C (%)", "ST (C)", "Drops", "Wait (s)", "RT (F)", "RH (%)", "Ramp (s)", "RPM", "Accel (RPM/s)", "Time (s)", "Mobility", "On/Off", "Vt", "S.T.S") -> (→"Transformer \nHeaders":string[])
